vi "SCA-RT_new.vi"() -> ()   [LabVIEW 2016]
uses:
  controls/SCA states.ctl
  control vi/controls/Gate Valve Readback.ctl
  controls/Vertical Rod states.ctl
  controls/Horizontal Rod states.ctl
  controls/GP307 cluster.ctl
  controls/SCA commands.ctl
  controls/SCA Bypass control.ctl
  controls/SCA broadcast status.ctl
  <vilib>/Platform/TimedLoop/XDataNode/timing_clust.ctl
  <vilib>/Platform/TimedLoop/XDataNode/nitl_modes.ctl
  <vilib>/Platform/TimedLoop/XDataNode/wakeup.ctl
  controls/Encoder bit cluster.ctl
  <vilib>/Analysis/baseanly.llb/Mean (DBL).vi
  <vilib>/Instr/_visa.llb/VISA Configure Serial Port (Instr).vi
  <vilib>/Motion/Express/_s/nimc.fb.straightLineMove.startStraightLineMove.axis.modeRelative.0.vi
  <vilib>/Platform/TimedLoop/XDataNode/loadnilvce.vi
  <vilib>/Motion/BlockNode/FB.NIMotion.xnode
  <vilib>/Platform/TimedLoop/XDataNode/XDataNode.xnode
  <vilib>/Platform/TimedLoop/XDataNode/XDNodeRunTimeDep.lvlib
  <vilib>/Analysis/NI_AALBase.lvlib
  <vilib>/NI_Real-Time Target Support.lvlib
panel:
  in  "New sample":i8=1
  in  "Step Window Radius":u8=1
  in  "Rollover Sample":i16=64
  in  "Encoder Offset":i16=160
  out "Bypass error":errorcluster
  out "HV Readback error":errorcluster
  out "SCA command monitor error":errorcluster
  in  "Insert Rod Bypass":bool
  in  "Retract Rod Bypass":bool
  in  "Sample Rod Bypass":bool
  in  "Wheel GV Bypass":bool
  out "Bypass Control":T1
  out "Immersion Lens I set":dbl
  out "Immersion Lens V Set":dbl
  out "SCA Command":T2=enum."Retract insert rod"
  out "Encoder error":errorcluster
  out "Convectron readback error":errorcluster
  out "HV Control error":errorcluster
  out "Rotate Wheel error":errorcluster
  out "Ion Source Vac Cluster":T3
  out "Bellows Vac Cluster":T3
  out "SCA-cRIO error":errorcluster
  out "Insert Rod Status":T4
  out "Retract Rod Status":T4
  out "Sample Rod status":T5
  out "Wheel GV":T6
  out "Raw bits":bool[](array[boolean])
  out "Converted bits":bool[](array[boolean])
  out "Immersion Lens I read":dbl format="%0.2f"
  out "Immersion Lens V read":dbl format="%0.2f"
  out "SCA next state":T7
  out "Extractor I read":dbl
  out "Extractor V read":dbl
  out "Extractor V set":dbl
  out "Cathode V read":dbl
  out "Cathode I read":dbl
  out "Cathode V set":dbl
  out "New Move":dbl
  out "Encoder Destination":dbl
  out "In Range?":bool
  out "Window Limit 2":u32
  out "Window Limit 1":u32
  out "Encoder position":u16
  out "action":string
  out "Vac Readback error":errorcluster
  out "Sample Wheel Convectron":string
  out "Sample Rod UP sensor":bool
  out "Sample Rod DOWN sensor":bool
  out "Rotation done":bool
  out "Insert Rod IN sensor":bool
  out "Insert Rod OUT sensor":bool
  out "Retract Rod IN sensor":bool
  out "Retract Rod OUT sensor":bool
  out "Sensor error":errorcluster
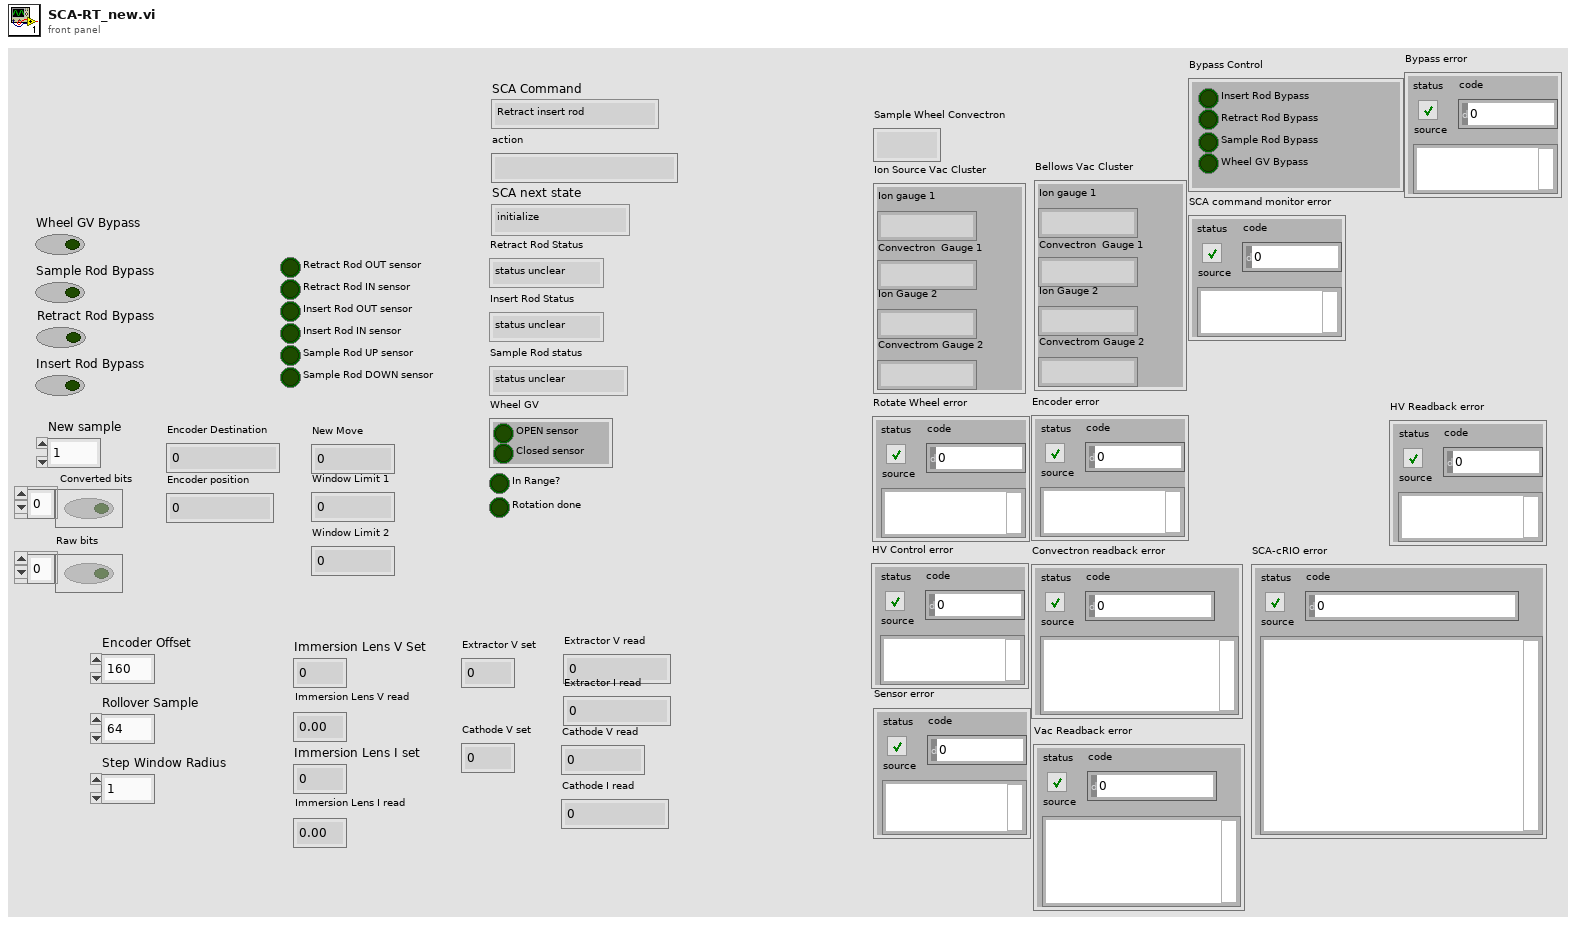
[diagram p1: front panel]
types:
  T1 = typedef "SCA Bypass control.ctl" = cluster{"Insert Rod Bypass":bool, "Retract Rod Bypass":bool, "Sample Rod Bypass":bool, "Wheel GV Bypass":bool}
  T2 = typedef "SCA commands.ctl" = enum16{"Wait", "Shutdown", "Retract insert rod", "Insert insert rod", "Retract retract rod", "Insert retract rod", "Retract sample rod", "Insert sample rod", "Open wheel GV", "Close wheel GV", "Open ion source GV", "Close ion source GV", "Pump out source", "Vent source", "Rotate wheel randomly", "Rotate wheel", "Start random sample change", "Start sample change"}
  T3 = typedef "GP307 cluster.ctl" = cluster{"Ion gauge 1":string, "Convectron  Gauge 1 ":string, "Ion Gauge 2":string, "Convectrom Gauge 2":string}
  T4 = typedef "Horizontal Rod states.ctl" = enum16{"status unclear", "rod in", "rod out"}
  T5 = typedef "Vertical Rod states.ctl" = enum16{"status unclear", "rod down", "rod up"}
  T6 = typedef "Gate Valve Readback.ctl" = cluster{"OPEN sensor":bool, "Closed sensor":bool}
  T7 = typedef "SCA states.ctl" = enum16{"initialize", "wait", "change sample start", "change sample", "check position", "rotate wheel", "sample change complete", "sample rod up", "sample rod down", "retract rod in", "retract rod out", "insert rod in", "insert rod out", "wheel GV open", "wheel GV close", "vent source", "pump source", "shutdown"}
  T8 = typedef "SCA broadcast status.ctl" = enum16{"Waiting", "Changing samples", "Sample change complete", "Failure"}
  T9 = typedef "GV states.ctl" = enum16{"status unclear", "closed", "open"}
  T10 = typedef "XDNodeRunTimeDep.lvlib/timing_clust.ctl" = cluster{"Expected End [f-1]":u64, "Actual End [f-1]":u64, "Finished Late? [f-1]":bool, "Expected End [i-1]":u64, "Actual End [i-1]":u64, "Finished Late? [i-1]":bool, "Expected Start [i]":u64, "Actual Start [i]":u64, "Expected Start [f]":u64, "Actual Start [f]":u64, "Source Name":string, "Structure Name":string, "Period":i64, "Deadline":i64, "Offset":i64, "Start":i64, "Priority":i32, "Timeout":i32, "Mode":T11, "Wakeup Reason":T12, "Error":errorcluster, "Source Type":string, "Secondary Source Type":string, "Global End Time":u64, "Global Start Time":u64, "Frame Duration":u64, "Iteration Duration":u64, "Assigned CPU":i32, "I/O Scan Engine Mode":u32}
  T11 = typedef "XDNodeRunTimeDep.lvlib/nitl_modes.ctl" = enum32{"No Change", "Process missed periods, maintain original phase", "Discard missed periods, maintain original phase", "Process missed periods, ignore original phase", "Discard missed periods, ignore original phase"}
  T12 = typedef "XDNodeRunTimeDep.lvlib/wakeup.ctl" = enum32{"Normal", "Aborted", "Asynchronous wakeup", "Timing source error", "Timed loop error", "Timeout"}
  T13 = typedef "Encoder bit cluster.ctl" = cluster{"MSB":bool, "13th bit":bool, "12th bit":bool, "11th bit":bool, "10th bit":bool, "9th bit":bool, "8th bit":bool, "7th bit":bool, "6th bit":bool, "5th bit":bool, "4th bit":bool, "3rd bit":bool, "2nd bit":bool, "LSB":bool}
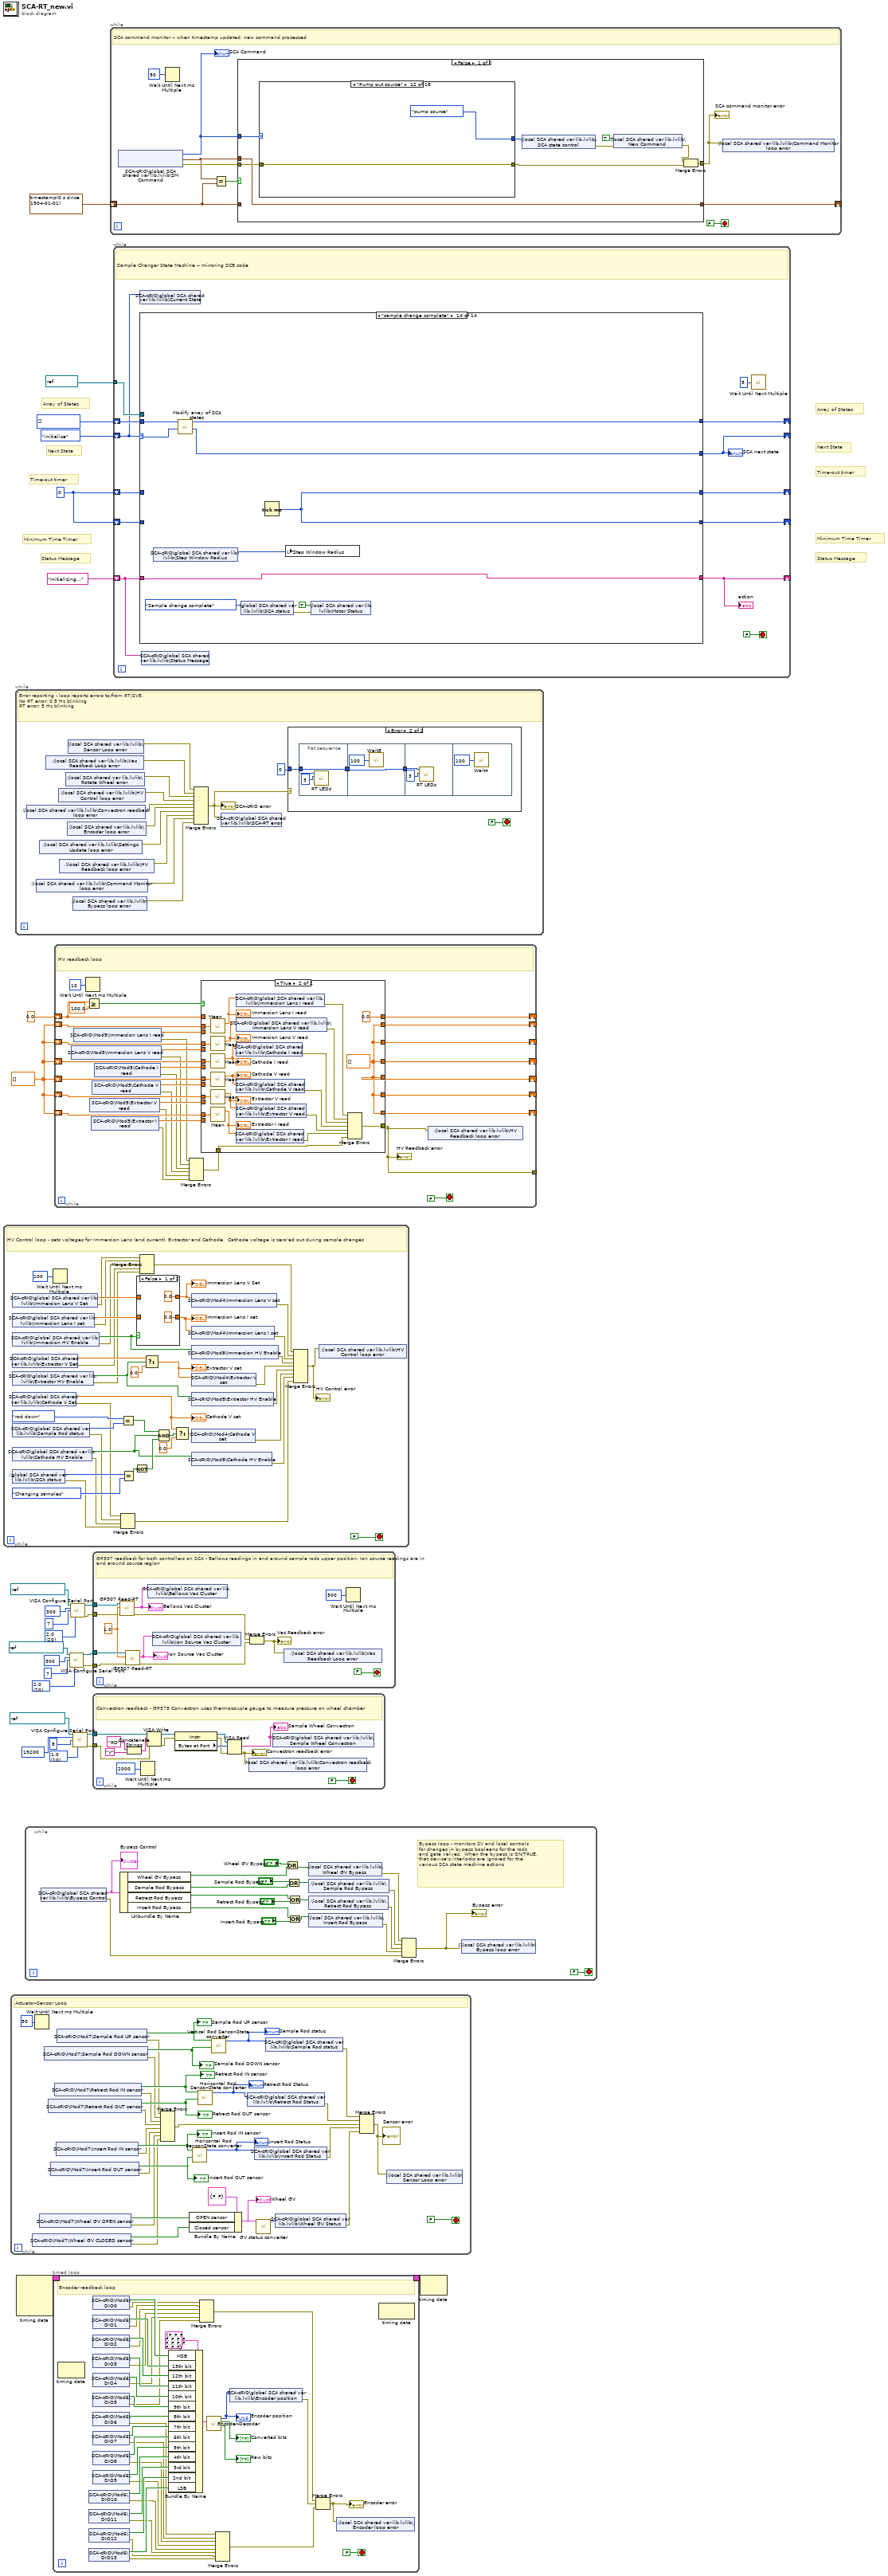
[diagram p0: block diagram]
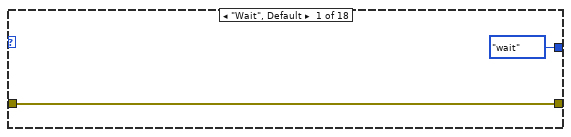
[diagram p2: hidden frame]
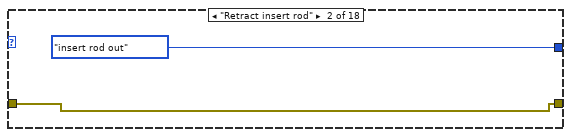
[diagram p3: hidden frame]
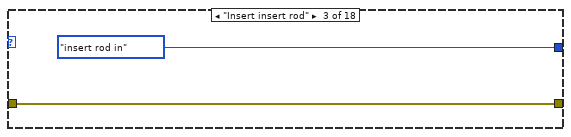
[diagram p4: hidden frame]
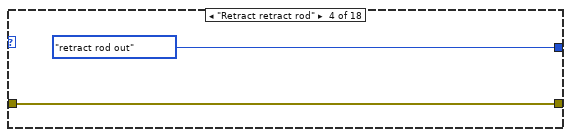
[diagram p5: hidden frame]
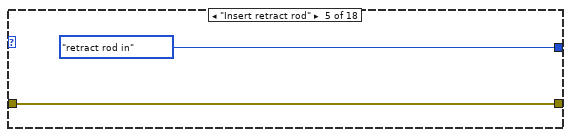
[diagram p6: hidden frame]
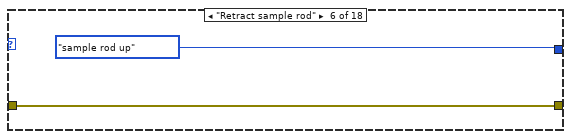
[diagram p7: hidden frame]
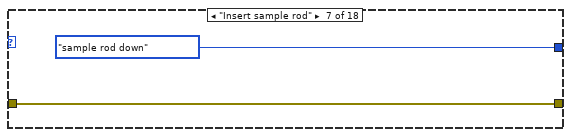
[diagram p8: hidden frame]
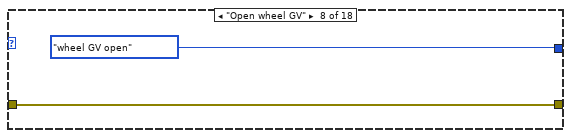
[diagram p9: hidden frame]
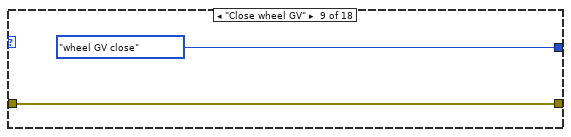
[diagram p10: hidden frame]
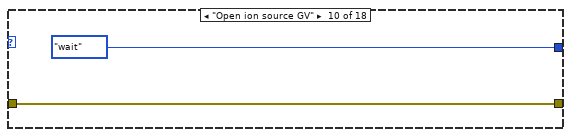
[diagram p11: hidden frame]
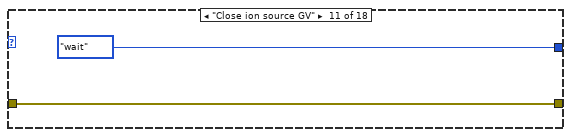
[diagram p12: hidden frame]
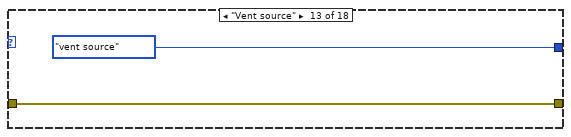
[diagram p13: hidden frame]
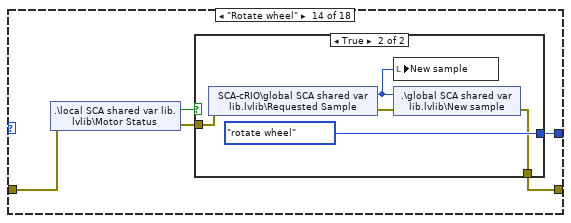
[diagram p14: hidden frame]
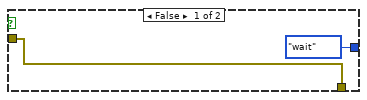
[diagram p15: hidden frame]
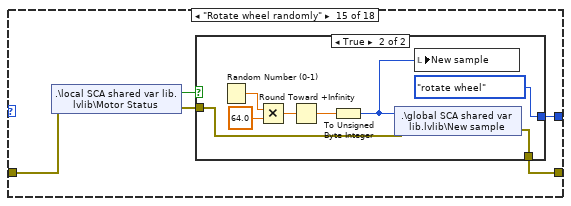
[diagram p16: hidden frame]
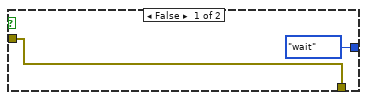
[diagram p17: hidden frame]
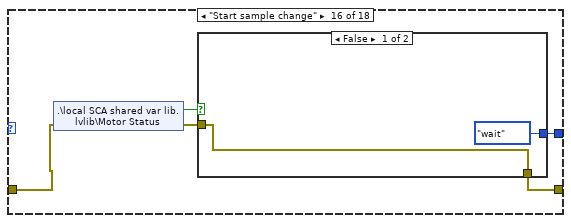
[diagram p18: hidden frame]
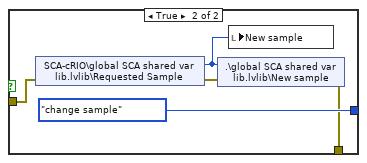
[diagram p19: hidden frame]
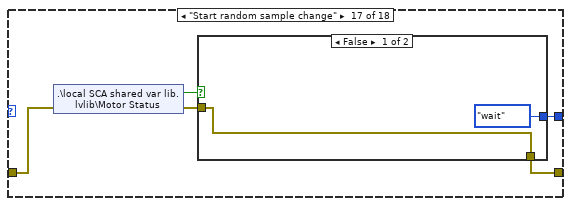
[diagram p20: hidden frame]
diagram:
  w4 = u32 0
  w6 = T7[] [] items=["initialize", "wait", "change sample start", "change sample", "check position", "rotate wheel", "sample change complete", "sample rod up", "sample rod down", "retract rod in", "retract rod out", "insert rod in", "insert rod out", "wheel GV open", "wheel GV close", "vent source", "pump source", "shutdown"]
  w22 = u16 20 items=["1.0"=10, "1.5"=15, "2.0"=20] ("stop bits (10: 1 bit)")
  w26 = u16 10 items=["1.0"=10, "1.5"=15, "2.0"=20] ("stop bits (10: 1 bit)")
  w16 = u16 20 items=["1.0"=10, "1.5"=15, "2.0"=20] ("stop bits (10: 1 bit)")
  w27 = dbl[] []
  # "Status Message"
  # "Array of States"
  # "Next State"
  # "Time-out timer"
  # "Minimum Time Timer"
  # "Status Message"
  # "Array of States"
  # "Next State"
  # "Time-out timer"
  # "Minimum Time Timer"
  n1 = while {
    stop <- FALSE stop-if-true
    # "HV Control loop - sets voltages for Immersion Lens (and current), Extractor and Cathode.  Cathode voltage is zero'ed out during sample changes"
    n2 = shared-variable "SCA-cRIO\\global SCA shared var lib.lvlib\\Immersion Lens V Set"() -> (w61:dbl, error out=w47:errorcluster)  [unwired: 1 in]
    n3 = shared-variable "SCA-cRIO\\global SCA shared var lib.lvlib\\Immersion Lens I set"() -> (w59:dbl, error out=w46:errorcluster)  [unwired: 1 in]
    n4 = shared-variable "SCA-cRIO\\global SCA shared var lib.lvlib\\Immersion HV Enable"() -> (w52:bool, error out=w45:errorcluster)  [unwired: 1 in]
    n5 = shared-variable "SCA-cRIO\\global SCA shared var lib.lvlib\\Extractor V Set"() -> (w57:dbl, error out=w44:errorcluster)  [unwired: 1 in]
    n6 = shared-variable "SCA-cRIO\\global SCA shared var lib.lvlib\\Extractor HV Enable"() -> (w51:bool, error out=w43:errorcluster)  [unwired: 1 in]
    n7 = shared-variable "SCA-cRIO\\global SCA shared var lib.lvlib\\Cathode V Set"() -> (w67:dbl, error out=w39:errorcluster)  [unwired: 1 in]
    "Cathode V set" <- w67
    n8 = shared-variable "SCA-cRIO\\global SCA shared var lib.lvlib\\Sample Rod status"() -> (w63:T5, error out=w40:errorcluster)  [unwired: 1 in]
    n9 = shared-variable "SCA-cRIO\\global SCA shared var lib.lvlib\\Cathode HV Enable"() -> (w53:bool, error out=w41:errorcluster)  [unwired: 1 in]
    n10 = shared-variable ".\\global SCA shared var lib.lvlib\\SCA status"() -> (w49:T8, error out=w42:errorcluster)  [unwired: 1 in]
    n11 = Wait Until Next ms Multiple(millisecond multiple=u32 100) -> ()  [unwired: 1 out]
    n12 = Equal?(x=Vertical_Rod_states."rod down", y=w63) -> (x = y?=w64:bool)
    n13 = Merge Errors(w39, w40, w41, w42) -> (w31:errorcluster)
    n14 = Equal?(x=w49, y=SCA_broadcast_status."Changing samples") -> (x = y?=w48:bool)
    n15 = Not(x=w48) -> (.not. x?=w54:bool)
    n16 = case shown="False" w52 {
      tunnel: [0.0 ("Double") w74] -> w60
      tunnel: w61 -> [_ w74]
      tunnel: w59 -> [_ w73]
      tunnel: [0.0 ("Double") w73] -> w58
      frame False {
      }
      frame True {
      }
    }
    "Immersion Lens V Set" <- w60
    "Immersion Lens I set" <- w58
    n17 = Merge Errors(w47, w46, w45, w44, w43) -> (w30:errorcluster)
    n18 = Select(t=w57, s=w51, f=0.0) -> (s? t:f=w56:dbl)
    "Extractor V set" <- w56
    n19 = Compound Arithmetic op=AND(w64, w53, w54) -> (w68:bool)
    n20 = Select(t=w67, s=w68, f=0.0) -> (s? t:f=w65:dbl)
    n21 = shared-variable "SCA-cRIO\\Mod4\\Immersion Lens V set"(w60) -> (error out=w36:errorcluster)  [unwired: 1 in]
    n22 = shared-variable "SCA-cRIO\\Mod4\\Immersion Lens I set"(w58) -> (error out=w37:errorcluster)  [unwired: 1 in]
    n23 = shared-variable "SCA-cRIO\\Mod8\\Immersion HV Enable"(w52) -> (error out=w38:errorcluster)  [unwired: 1 in]
    n24 = shared-variable "SCA-cRIO\\Mod4\\Extractor V set"(w56) -> (error out=w35:errorcluster)  [unwired: 1 in]
    n25 = shared-variable "SCA-cRIO\\Mod8\\Extractor HV Enable"(w51) -> (error out=w34:errorcluster)  [unwired: 1 in]
    n26 = shared-variable "SCA-cRIO\\Mod4\\Cathode V set"(w65) -> (error out=w33:errorcluster)  [unwired: 1 in]
    n27 = shared-variable "SCA-cRIO\\Mod8\\Cathode HV Enable"(w53) -> (error out=w32:errorcluster)  [unwired: 1 in]
    n28 = Merge Errors(w30, w36, w37, w38, w35, w34, w33, w32, w31) -> (w29:errorcluster)
    "HV Control error" <- w29
    n29 = shared-variable ".\\local SCA shared var lib.lvlib\\HV Control loop error"(w29) -> ()  [unwired: 1 in, 1 out]
  }
  n30 = while {
    stop <- FALSE ("stop") stop-if-true
    # "Actuator-Sensor Loop"
    n31 = shared-variable "SCA-cRIO\\Mod7\\Wheel GV CLOSED sensor"() -> (w100:bool, error out=w79:errorcluster)  [unwired: 1 in]
    n32 = Wait Until Next ms Multiple(millisecond multiple=u32 50) -> ()  [unwired: 1 out]
    n33 = shared-variable "SCA-cRIO\\Mod7\\Wheel GV OPEN sensor"() -> (w99:bool, error out=w78:errorcluster)  [unwired: 1 in]
    n34 = shared-variable "SCA-cRIO\\Mod7\\Sample Rod DOWN sensor"() -> (w96:bool, error out=w82:errorcluster)  [unwired: 1 in]
    "Sample Rod DOWN sensor" <- w96
    n35 = shared-variable "SCA-cRIO\\Mod7\\Retract Rod OUT sensor"() -> (w93:bool, error out=w80:errorcluster)  [unwired: 1 in]
    "Retract Rod OUT sensor" <- w93
    n36 = shared-variable "SCA-cRIO\\Mod7\\Insert Rod OUT sensor"() -> (w91:bool, error out=w77:errorcluster)  [unwired: 1 in]
    "Insert Rod OUT sensor" <- w91
    n37 = shared-variable "SCA-cRIO\\Mod7\\Retract Rod IN sensor"() -> (w94:bool, error out=w81:errorcluster)  [unwired: 1 in]
    "Retract Rod IN sensor" <- w94
    n38 = shared-variable "SCA-cRIO\\Mod7\\Insert Rod IN sensor"() -> (w92:bool, error out=w76:errorcluster)  [unwired: 1 in]
    "Insert Rod IN sensor" <- w92
    n39 = shared-variable "SCA-cRIO\\Mod7\\Sample Rod UP sensor"() -> (w97:bool, error out=w83:errorcluster)  [unwired: 1 in]
    "Sample Rod UP sensor" <- w97
    n40 = Merge Errors(w83, w82, w81, w80, w76, w77, w78, w79) -> (w75:errorcluster)
    n41 = Bundle By Name(cluster=T6 {"OPEN sensor"=FALSE, "Closed sensor"=FALSE} ("Gate Valve"), "OPEN sensor"=w99, "Closed sensor"=w100) -> (w102:T6)
    "Wheel GV" <- w102
    n42 = call "Horizontal Rod Sensor-State converter.vi"("IN Sensor"=w92, "OUT Sensor"=w91) -> ("Status"=w90:T4)  [unwired: 8 in]
    "Insert Rod Status" <- w90
    n43 = call "Horizontal Rod Sensor-State converter.vi"("IN Sensor"=w94, "OUT Sensor"=w93) -> ("Status"=w89:T4)  [unwired: 8 in]
    "Retract Rod Status" <- w89
    n44 = call "Vertical Rod Sensor-State converter.vi"("UP Sensor"=w97, "DOWN Sensor"=w96) -> ("Status"=w95:T5)  [unwired: 8 in]
    "Sample Rod status" <- w95
    n45 = shared-variable "SCA-cRIO\\global SCA shared var lib.lvlib\\Retract Rod Status"(w89) -> (error out=w86:errorcluster)  [unwired: 1 in]
    n46 = shared-variable "SCA-cRIO\\global SCA shared var lib.lvlib\\Insert Rod Status"(w90) -> (error out=w85:errorcluster)  [unwired: 1 in]
    n47 = call "GV status converter.vi"("Gate Valve"=w102) -> ("GV Status"=w98:T9)  [unwired: 10 in]
    n48 = shared-variable "SCA-cRIO\\global SCA shared var lib.lvlib\\Sample Rod status"(w95) -> (error out=w87:errorcluster)  [unwired: 1 in]
    n49 = shared-variable "SCA-cRIO\\global SCA shared var lib.lvlib\\Wheel GV Status"(w98) -> (error out=w84:errorcluster)  [unwired: 1 in]
    n50 = Merge Errors(w87, w86, w75, w85, w84) -> (w88:errorcluster)
    "Sensor error" <- w88
    n51 = shared-variable ".\\local SCA shared var lib.lvlib\\Sensor Loop error"(w88) -> ()  [unwired: 1 in, 1 out]
  }
  n52 = while {
    stop <- FALSE stop-if-true
    # "Error reporting - loop reports errors to/from RT/SVE. \nNo RT error: 0.5 Hz blinking\nRT error: 5 Hz blinking"
    n53 = shared-variable ".\\local SCA shared var lib.lvlib\\Convectron readback loop error"() -> (w110:errorcluster)  [unwired: 1 in, 1 out]
    n54 = shared-variable ".\\local SCA shared var lib.lvlib\\Command Monitor loop error"() -> (w106:errorcluster)  [unwired: 1 in, 1 out]
    n55 = shared-variable ".\\local SCA shared var lib.lvlib\\Settings Update loop error"() -> (w108:errorcluster)  [unwired: 1 in, 1 out]
    n56 = shared-variable ".\\local SCA shared var lib.lvlib\\Vac Readback Loop error"() -> (w115:errorcluster)  [unwired: 1 in, 1 out]
    n57 = shared-variable ".\\local SCA shared var lib.lvlib\\HV Control loop error"() -> (w111:errorcluster)  [unwired: 1 in, 1 out]
    n58 = shared-variable ".\\local SCA shared var lib.lvlib\\HV Readback loop error"() -> (w107:errorcluster)  [unwired: 1 in, 1 out]
    n59 = shared-variable ".\\local SCA shared var lib.lvlib\\Rotate Wheel error"() -> (w112:errorcluster)  [unwired: 1 in, 1 out]
    n60 = shared-variable ".\\local SCA shared var lib.lvlib\\Encoder loop error"() -> (w109:errorcluster)  [unwired: 1 in, 1 out]
    n61 = shared-variable ".\\local SCA shared var lib.lvlib\\Sensor Loop error"() -> (w116:errorcluster)  [unwired: 1 in, 1 out]
    n62 = shared-variable ".\\local SCA shared var lib.lvlib\\Bypass loop error"() -> (w105:errorcluster)  [unwired: 1 in, 1 out]
    n63 = Merge Errors(w116, w115, w112, w111, w110, w109, w108, w107, w106, w105) -> (w114:errorcluster)
    "SCA-cRIO error" <- w114
    n64 = shared-variable "SCA-cRIO\\global SCA shared var lib.lvlib\\SCA-RT error"(w114) -> ()  [unwired: 1 in, 1 out]
    n65 = case shown="Error" w114 {
      tunnel: 0 -> [w120 w128]
      frame No Error {
        n66 = flat-sequence {
          tunnel: w120 -> [w121]
          tunnel: [w121] -> w118
          tunnel: [w123] -> w119
          tunnel: w118 -> [w123]
          tunnel: w119 -> [w125]
          frame #0 {
            n67 = call <vilib>:"RT LEDs.vi"("State"=3, "LED Num"=w121) -> ()  [unwired: 4 in, 2 out]
          }
          frame #1 {
            n68 = call "Wait"("Count(mSec)"=u16 1000) -> ()  [unwired: 1 out]
          }
          frame #2 {
            n69 = call <vilib>:"RT LEDs.vi"("State"=3, "LED Num"=w125) -> ()  [unwired: 4 in, 2 out]
          }
          frame #3 {
            n70 = call "Wait2"("Count(mSec)"=u16 1000) -> ()  [unwired: 1 out]
          }
        }
      }
      frame Error {
        n71 = flat-sequence {
          tunnel: [w131] -> w130
          tunnel: w128 -> [w131]
          tunnel: w130 -> [w133]
          tunnel: [w133] -> w129
          tunnel: w129 -> [w135]
          frame #0 {
            n72 = call <vilib>:"RT LEDs.vi"("State"=3, "LED Num"=w131) -> ()  [unwired: 4 in, 2 out]
          }
          frame #1 {
            n73 = call "Wait3"("Count(mSec)"=u16 100) -> ()  [unwired: 1 out]
          }
          frame #2 {
            n74 = call <vilib>:"RT LEDs.vi"("State"=3, "LED Num"=w135) -> ()  [unwired: 4 in, 2 out]
          }
          frame #3 {
            n75 = call "Wait4"("Count(mSec)"=u16 100) -> ()  [unwired: 1 out]
          }
        }
      }
    }
  }
  n76 = node-c288() -> (w8:T10)  [unwired: 4 in]
  n77 = while {
    stop <- FALSE stop-if-true
    # "Bypass loop - monitors SV and local controls\nfor changes in bypass booleans for the rods \nand gate valves.  When the bypass is ON/TRUE,\nthat device's interlocks are ignored for the \nvarious SCA state machine actions"
    n78 = shared-variable "SCA-cRIO\\global SCA shared var lib.lvlib\\Bypass Control"() -> (w151:T1, error out=w139:errorcluster)  [unwired: 1 in]
    "Bypass Control" <- w151
    n79 = Unbundle By Name(w151) -> ("Wheel GV Bypass"=w148:bool, "Sample Rod Bypass"=w147:bool, "Retract Rod Bypass"=w146:bool, "Insert Rod Bypass"=w145:bool)
    n80 = Or(x="Wheel GV Bypass", y=w148) -> (x .or. y?=w155:bool)
    n81 = Or(x="Sample Rod Bypass", y=w147) -> (x .or. y?=w154:bool)
    n82 = Or(x=w146, y="Retract Rod Bypass") -> (x .or. y?=w152:bool)
    n83 = Or(x=w145, y="Insert Rod Bypass") -> (x .or. y?=w153:bool)
    n84 = shared-variable ".\\local SCA shared var lib.lvlib\\Wheel GV Bypass"(w155) -> (error out=w143:errorcluster)  [unwired: 1 in]
    n85 = shared-variable ".\\local SCA shared var lib.lvlib\\Sample Rod Bypass"(w154) -> (error out=w142:errorcluster)  [unwired: 1 in]
    n86 = shared-variable ".\\local SCA shared var lib.lvlib\\Retract Rod Bypass"(w152) -> (error out=w141:errorcluster)  [unwired: 1 in]
    n87 = shared-variable ".\\local SCA shared var lib.lvlib\\Insert Rod Bypass"(w153) -> (error out=w140:errorcluster)  [unwired: 1 in]
    n88 = Merge Errors(w143, w142, w141, w140, w139) -> (w138:errorcluster)
    "Bypass error" <- w138
    n89 = shared-variable ".\\local SCA shared var lib.lvlib\\Bypass loop error"(w138) -> ()  [unwired: 1 in, 1 out]
  }
  n90 = timed-loop {
    timing: w8 -> [_]
    timing-out: [_] -> w7
    stop <- FALSE stop-if-true
    # "Encoder readback loop"
    n91 = node-c288() -> ()  [unwired: 1 in, 1 out]
    n92 = shared-variable "SCA-cRIO\\Mod6\\DIO10"() -> (w187:bool, error out=w170:errorcluster)  [unwired: 1 in]
    n93 = shared-variable "SCA-cRIO\\Mod6\\DIO11"() -> (w186:bool, error out=w171:errorcluster)  [unwired: 1 in]
    n94 = shared-variable "SCA-cRIO\\Mod6\\DIO12"() -> (w185:bool, error out=w172:errorcluster)  [unwired: 1 in]
    n95 = shared-variable "SCA-cRIO\\Mod6\\DIO13"() -> (w184:bool, error out=w173:errorcluster)  [unwired: 1 in]
    n96 = shared-variable "SCA-cRIO\\Mod6\\DIO0"() -> (w193:bool, error out=w164:errorcluster)  [unwired: 1 in]
    n97 = shared-variable "SCA-cRIO\\Mod6\\DIO1"() -> (w192:bool, error out=w163:errorcluster)  [unwired: 1 in]
    n98 = shared-variable "SCA-cRIO\\Mod6\\DIO2"() -> (w183:bool, error out=w162:errorcluster)  [unwired: 1 in]
    n99 = shared-variable "SCA-cRIO\\Mod6\\DIO3"() -> (w182:bool, error out=w161:errorcluster)  [unwired: 1 in]
    n100 = shared-variable "SCA-cRIO\\Mod6\\DIO4"() -> (w191:bool, error out=w160:errorcluster)  [unwired: 1 in]
    n101 = shared-variable "SCA-cRIO\\Mod6\\DIO5"() -> (w190:bool, error out=w159:errorcluster)  [unwired: 1 in]
    n102 = shared-variable "SCA-cRIO\\Mod6\\DIO6"() -> (w189:bool, error out=w166:errorcluster)  [unwired: 1 in]
    n103 = shared-variable "SCA-cRIO\\Mod6\\DIO7"() -> (w176:bool, error out=w167:errorcluster)  [unwired: 1 in]
    n104 = shared-variable "SCA-cRIO\\Mod6\\DIO8"() -> (w188:bool, error out=w168:errorcluster)  [unwired: 1 in]
    n105 = shared-variable "SCA-cRIO\\Mod6\\DIO9"() -> (w181:bool, error out=w169:errorcluster)  [unwired: 1 in]
    n106 = Bundle By Name(cluster=T13 {"MSB"=FALSE, "13th bit"=FALSE, "12th bit"=FALSE, "11th bit"=FALSE, "10th bit"=FALSE, "9th bit"=FALSE, "8th bit"=FALSE, "7th bit"=FALSE, "6th bit"=FALSE, "5th bit"=FALSE, "4th bit"=FALSE, "3rd bit"=FALSE, "2nd bit"=FALSE, "LSB"=FALSE} ("Cluster"), "MSB"=w193, "13th bit"=w192, "12th bit"=w183, "11th bit"=w182, "10th bit"=w191, "9th bit"=w190, "8th bit"=w189, "7th bit"=w176, "6th bit"=w188, "5th bit"=w181, "4th bit"=w187, "3rd bit"=w186, "2nd bit"=w185, "LSB"=w184) -> (w195:T13)
    n107 = Merge Errors(w164, w163, w162, w161, w160, w159) -> (w158:errorcluster)
    n108 = call "Encoder-Decoder.vi"("Encoder data"=w195) -> ("Raw bits"=→"Raw bits":bool[], "Converted bits"=→"Converted bits":bool[], "Encoder position"=w180:u16)  [unwired: 8 in]
    "Encoder position" <- w180
    n109 = Merge Errors(w166, w167, w168, w169, w170, w171, w172, w173) -> (w165:errorcluster)
    n110 = shared-variable "SCA-cRIO\\global SCA shared var lib.lvlib\\Encoder position"(w180) -> (error out=w174:errorcluster)  [unwired: 1 in]
    n111 = Merge Errors(w158, w174, w165) -> (w175:errorcluster)
    "Encoder error" <- w175
    n112 = shared-variable ".\\local SCA shared var lib.lvlib\\Encoder loop error"(w175) -> ()  [unwired: 1 in, 1 out]
    n113 = node-c288() -> ()  [unwired: 1 in, 1 out]
  }
  n114 = while {
    shift-right: [w222] -> _
    shift-left: 0.0 ("AI1") -> [w225]
    shift-right: [w220] -> _
    shift-left: w27 -> [w219]
    shift-right: [w221] -> _
    shift-left: w27 -> [w218]
    shift-right: [w216] -> _
    shift-left: w27 -> [w215]
    shift-right: [w213] -> _
    shift-left: w27 -> [w212]
    shift-right: [w207] -> _
    shift-left: w27 -> [w210]
    shift-right: [w206] -> _
    shift-left: w27 -> [w211]
    tunnel: [w198] -> _
    stop <- FALSE stop-if-true
    # "HV readback loop"
    n115 = shared-variable "SCA-cRIO\\Mod5\\Immersion Lens V read"() -> (w208:dbl, error out=w204:errorcluster)  [unwired: 1 in]
    n116 = shared-variable "SCA-cRIO\\Mod5\\Immersion Lens I read"() -> (w209:dbl, error out=w205:errorcluster)  [unwired: 1 in]
    n117 = Wait Until Next ms Multiple(millisecond multiple=u32 10) -> ()  [unwired: 1 out]
    n118 = Greater Or Equal?(x=w225, y=100.0) -> (x >= y?=w223:bool)
    n119 = shared-variable "SCA-cRIO\\Mod5\\Extractor V read"() -> (w217:dbl, error out=w201:errorcluster)  [unwired: 1 in]
    n120 = shared-variable "SCA-cRIO\\Mod5\\Extractor I read"() -> (w214:dbl, error out=w200:errorcluster)  [unwired: 1 in]
    n121 = shared-variable "SCA-cRIO\\Mod5\\Cathode V read"() -> (w227:dbl, error out=w202:errorcluster)  [unwired: 1 in]
    n122 = shared-variable "SCA-cRIO\\Mod5\\Cathode I read"() -> (w226:dbl, error out=w203:errorcluster)  [unwired: 1 in]
    n123 = Merge Errors(w205, w204, w203, w202, w201, w200) -> (w199:errorcluster)
    n124 = case shown="True" w223 {
      tunnel: w227 -> [w246 _]
      tunnel: w226 -> [w247 _]
      tunnel: w225 -> [w250 _]
      tunnel: [w249 0.0 ("AI1")] -> w222
      tunnel: [w248 w262] -> w221
      tunnel: [w245 w262] -> w220
      tunnel: w219 -> [w244 w270]
      tunnel: w218 -> [w243 w271]
      tunnel: w217 -> [w242 _]
      tunnel: [w241 w262] -> w216
      tunnel: w215 -> [w240 w269]
      tunnel: w214 -> [w239 _]
      tunnel: [w238 w262] -> w213
      tunnel: w212 -> [w237 w268]
      tunnel: w211 -> [w236 w261]
      tunnel: w210 -> [w235 w260]
      tunnel: w209 -> [w234 _]
      tunnel: w208 -> [w233 _]
      tunnel: [w232 w262] -> w207
      tunnel: [w231 w262] -> w206
      tunnel: w199 -> [w230 w257]
      tunnel: [w230 w251] -> w198
      frame False {
        n125 = Build Array (concatenate)(w234, w235) -> (w232:dbl[])
        n126 = Build Array (concatenate)(w233, w236) -> (w231:dbl[])
        n127 = Build Array (concatenate)(w247, w243) -> (w248:dbl[])
        n128 = Build Array (concatenate)(w246, w244) -> (w245:dbl[])
        n129 = Build Array (concatenate)(w242, w240) -> (w241:dbl[])
        n130 = Build Array (concatenate)(w239, w237) -> (w238:dbl[])
        n131 = Increment(x=w250) -> (x+1=w249:dbl)
      }
      frame True {
        w262 = dbl[] []
        n132 = call-poly <vilib>:"Mean.vi"("X"=w260) -> ("mean"=w259:dbl)  [unwired: 1 out]
        "Immersion Lens I read" <- w259
        n133 = call-poly <vilib>:"Mean.vi"("X"=w261) -> ("mean"=w263:dbl)  [unwired: 1 out]
        "Immersion Lens V read" <- w263
        n134 = call-poly <vilib>:"Mean.vi"("X"=w271) -> ("mean"=w267:dbl)  [unwired: 1 out]
        "Cathode I read" <- w267
        n135 = call-poly <vilib>:"Mean.vi"("X"=w270) -> ("mean"=w266:dbl)  [unwired: 1 out]
        "Cathode V read" <- w266
        n136 = call-poly <vilib>:"Mean.vi"("X"=w269) -> ("mean"=w265:dbl)  [unwired: 1 out]
        "Extractor V read" <- w265
        n137 = call-poly <vilib>:"Mean.vi"("X"=w268) -> ("mean"=w264:dbl)  [unwired: 1 out]
        "Extractor I read" <- w264
        n138 = shared-variable "SCA-cRIO\\global SCA shared var lib.lvlib\\Immersion Lens I read"(w259) -> (error out=w258:errorcluster)  [unwired: 1 in]
        n139 = shared-variable "SCA-cRIO\\global SCA shared var lib.lvlib\\Immersion Lens V read"(w263) -> (error out=w256:errorcluster)  [unwired: 1 in]
        n140 = shared-variable "SCA-cRIO\\global SCA shared var lib.lvlib\\Cathode I read"(w267) -> (error out=w255:errorcluster)  [unwired: 1 in]
        n141 = shared-variable "SCA-cRIO\\global SCA shared var lib.lvlib\\Cathode V read"(w266) -> (error out=w254:errorcluster)  [unwired: 1 in]
        n142 = shared-variable "SCA-cRIO\\global SCA shared var lib.lvlib\\Extractor V read"(w265) -> (error out=w253:errorcluster)  [unwired: 1 in]
        n143 = shared-variable "SCA-cRIO\\global SCA shared var lib.lvlib\\Extractor I read"(w264) -> (error out=w252:errorcluster)  [unwired: 1 in]
        n144 = Merge Errors(w258, w256, w255, w254, w253, w252, w257) -> (w251:errorcluster)
      }
    }
    "HV Readback error" <- w198
    n145 = shared-variable ".\\local SCA shared var lib.lvlib\\HV Readback loop error"(w198) -> ()  [unwired: 1 in, 1 out]
  }
  n146 = call-poly "VISA Configure Serial Port"("VISA resource name"=refnum<visa-resource-name> "ASRL2::INSTR", "baud rate (9600)"=u32 300, "data bits (8)"=u16 7, "stop bits (10: 1 bit)"=w16) -> ("VISA resource name out"=w17:refnum<visa-resource-name>, "error out"=w10:errorcluster)  [unwired: 10 in]
  n147 = call-poly "VISA Configure Serial Port"("VISA resource name"=refnum<visa-resource-name> "ASRL4::INSTR", "baud rate (9600)"=u32 300, "data bits (8)"=u16 7, "stop bits (10: 1 bit)"=w22) -> ("VISA resource name out"=w23:refnum<visa-resource-name>, "error out"=w11:errorcluster)  [unwired: 10 in]
  n148 = call-poly "VISA Configure Serial Port"("VISA resource name"=refnum<visa-resource-name> "ASRL3::INSTR", "baud rate (9600)"=u32 19200, "data bits (8)"=u16 8, "stop bits (10: 1 bit)"=w26) -> ("VISA resource name out"=w12:refnum<visa-resource-name>, "error out"=w9:errorcluster)  [unwired: 10 in]
  n149 = while {
    tunnel: w17 -> [w278]
    tunnel: w23 -> [w281]
    tunnel: w11 -> [w274]
    tunnel: w10 -> [w273]
    stop <- FALSE ("stop 4") stop-if-true
    w277 = 1.0 ("Delay Time (s)")
    # "GP307 readback for both controllers on SCA - Bellows readings in and around sample rods upper position; Ion source readings are in and around source region"
    n150 = call "GP307 Read-RT.vi"("error in (no error)"=w274, "Delay Time (s)"=w277, "VISA Refnum in"=w281) -> ("error out"=w279:errorcluster, "GP307 output"=w280:T3)  [unwired: 6 in, 1 out]
    "Bellows Vac Cluster" <- w280
    n151 = call "GP307 Read-RT.vi"("error in (no error)"=w273, "Delay Time (s)"=w277, "VISA Refnum in"=w278) -> ("error out"=w275:errorcluster, "GP307 output"=w276:T3)  [unwired: 6 in, 1 out]
    "Ion Source Vac Cluster" <- w276
    n152 = shared-variable "SCA-cRIO\\global SCA shared var lib.lvlib\\Bellows Vac Cluster"(w280) -> ()  [unwired: 1 in, 1 out]
    n153 = shared-variable "SCA-cRIO\\global SCA shared var lib.lvlib\\Ion Source Vac Cluster"(w276) -> ()  [unwired: 1 in, 1 out]
    n154 = Merge Errors(w279, w275) -> (w282:errorcluster)
    "Vac Readback error" <- w282
    n155 = shared-variable ".\\local SCA shared var lib.lvlib\\Vac Readback Loop error"(w282) -> ()  [unwired: 1 in, 1 out]
    n156 = Wait Until Next ms Multiple(millisecond multiple=u32 500) -> ()  [unwired: 1 out]
  }
  n157 = while {
    tunnel: w12 -> [w291]
    tunnel: w9 -> [w285]
    stop <- FALSE ("stop 3") stop-if-true
    # "Convectron readback - GP375 Convectron uses thermocouple gauge to measure pressure on wheel chamber"
    n158 = Concatenate Strings("RD" ("write buffer 2"), "\r") -> (w298:string)
    n159 = Wait Until Next ms Multiple(millisecond multiple=u32 2000) -> ()  [unwired: 1 out]
    n160 = VISA Write(VISA resource name=w291, write buffer=w298, error in (no error)=w285) -> (VISA resource name out=w292:refnum<visa-resource-name>, error out=w288:errorcluster)  [unwired: 1 out]
    n161 = property class="Instr"(reference=w292, error in=w288) -> (reference out=w293:refnum<visa-resource-name>, error out=w287:errorcluster, "Bytes at Port"=w294:u32)
    n162 = VISA Read(VISA resource name=w293, byte count=w294, error in (no error)=w287) -> (read buffer=w289:string, error out=w286:errorcluster)  [unwired: 2 out]
    "Sample Wheel Convectron" <- w289
    "Convectron readback error" <- w286
    n163 = shared-variable ".\\local SCA shared var lib.lvlib\\Convectron readback loop error"(w286) -> ()  [unwired: 1 in, 1 out]
    n164 = shared-variable "SCA-cRIO\\global SCA shared var lib.lvlib\\Sample Wheel Convectron"(w289) -> ()  [unwired: 1 in, 1 out]
  }
  n165 = while {
    shift-right: [w305] -> _
    shift-left: timestamp(0 s since 1904-01-01) -> [w304]
    stop <- FALSE stop-if-true
    # "SCA command monitor -- when timestamp updated, new command processed"
    n166 = shared-variable "SCA-cRIO\\global SCA shared var lib.lvlib\\SM Command"() -> (w301:T2, error out=w300:errorcluster, w306:timestamp)  [unwired: 1 in]
    "SCA Command" <- w301
    n167 = Wait Until Next ms Multiple(millisecond multiple=u32 50) -> ()  [unwired: 1 out]
    n168 = Equal?(x=w306, y=w304) -> (x = y?=w307:bool)
    n169 = case shown="False" w307 {
      tunnel: w306 -> [w316 _]
      tunnel: [w316 w400] -> w305
      tunnel: w304 -> [_ w400]
      tunnel: w301 -> [w315 _]
      tunnel: w300 -> [w311 w399]
      tunnel: [w308 w399] -> w299
      frame False {
        n170 = case shown="\"Pump out source\"" w315 {
          tunnel: [SCA_states."wait" ("SC2 state") SCA_states."insert rod out" ("SC2 state") SCA_states."insert rod in" ("SC2 state") SCA_states."retract rod out" ("SC2 state") SCA_states."retract rod in" ("SC2 state") SCA_states."sample rod up" ("SC2 state") SCA_states."sample rod down" ("SC2 state") SCA_states."wheel GV open" ("SC2 state") SCA_states."wheel GV close" ("SC2 state") SCA_states."wait" ("SC2 state") SCA_states."wait" ("SC2 state") SCA_states."pump source" ("SC2 state") SCA_states."vent source" ("SC2 state") w347 w359 w374 w385 SCA_states."initialize" ("SC2 state")] -> w314
          tunnel: w311 -> [w318 w319 w321 w323 w325 w327 w329 w331 w333 w335 w337 w339 w341 w345 w357 w372 w384 w398]
          tunnel: [w318 w319 w321 w323 w325 w327 w329 w331 w333 w335 w337 w339 w341 w343 w355 w370 w383 w398] -> w310
          frame "Wait", Default {
          }
          frame "Retract insert rod" {
          }
          frame "Insert insert rod" {
          }
          frame "Retract retract rod" {
          }
          frame "Insert retract rod" {
          }
          frame "Retract sample rod" {
          }
          frame "Insert sample rod" {
          }
          frame "Open wheel GV" {
          }
          frame "Close wheel GV" {
          }
          frame "Open ion source GV" {
          }
          frame "Close ion source GV" {
          }
          frame "Pump out source" {
          }
          frame "Vent source" {
          }
          frame "Rotate wheel" {
            n171 = shared-variable ".\\local SCA shared var lib.lvlib\\Motor Status"(error in=w345) -> (w346:bool, error out=w344:errorcluster)
            n172 = case shown="True" w346 {
              tunnel: [SCA_states."wait" ("SC2 state") SCA_states."rotate wheel" ("SC2 state")] -> w347
              tunnel: w344 -> [w348 w353]
              tunnel: [w348 w351] -> w343
              frame False {
              }
              frame True {
                n173 = shared-variable "SCA-cRIO\\global SCA shared var lib.lvlib\\Requested Sample"(error in=w353) -> (w350:u8, error out=w352:errorcluster)
                n174 = local write "New sample"(w350) -> ()
                n175 = shared-variable ".\\global SCA shared var lib.lvlib\\New sample"(w350, error in=w352) -> (error out=w351:errorcluster)
              }
            }
          }
          frame "Rotate wheel randomly" {
            n176 = shared-variable ".\\local SCA shared var lib.lvlib\\Motor Status"(error in=w357) -> (w358:bool, error out=w356:errorcluster)
            n177 = case shown="True" w358 {
              tunnel: [SCA_states."wait" ("SC2 state") SCA_states."rotate wheel" ("SC2 state")] -> w359
              tunnel: w356 -> [w360 w364]
              tunnel: [w360 w363] -> w355
              frame False {
              }
              frame True {
                n178 = Random Number (0-1)() -> (number: 0 to 1=w367:dbl)
                n179 = Multiply(x=w367, y=64.0) -> (x*y=w365:dbl)
                n180 = Round Toward +Infinity(x=w365) -> (ceil(x): smallest int >= x=w368:dbl)
                n181 = To Unsigned Byte Integer(number=w368) -> (unsigned 8bit integer=w362:u8)
                n182 = shared-variable ".\\global SCA shared var lib.lvlib\\New sample"(w362, error in=w364) -> (error out=w363:errorcluster)
                n183 = local write "New sample"(w362) -> ()
              }
            }
          }
          frame "Start sample change" {
            n184 = shared-variable ".\\local SCA shared var lib.lvlib\\Motor Status"(error in=w372) -> (w373:bool, error out=w371:errorcluster)
            n185 = case shown="False" w373 {
              tunnel: [SCA_states."wait" ("SC2 state") SCA_states."change sample" ("SC2 state")] -> w374
              tunnel: w371 -> [w375 w380]
              tunnel: [w375 w378] -> w370
              frame False {
              }
              frame True {
                n186 = shared-variable "SCA-cRIO\\global SCA shared var lib.lvlib\\Requested Sample"(error in=w380) -> (w377:u8, error out=w379:errorcluster)
                n187 = shared-variable ".\\global SCA shared var lib.lvlib\\New sample"(w377, error in=w379) -> (error out=w378:errorcluster)
                n188 = local write "New sample"(w377) -> ()
              }
            }
          }
          frame "Start random sample change" {
            n189 = shared-variable ".\\local SCA shared var lib.lvlib\\Motor Status"(error in=w384) -> (w386:bool, error out=w382:errorcluster)
            n190 = case shown="False" w386 {
              tunnel: [SCA_states."wait" ("SC2 state") SCA_states."change sample" ("SC2 state")] -> w385
              tunnel: [w387 w391] -> w383
              tunnel: w382 -> [w387 w390]
              frame False {
              }
              frame True {
                n191 = Random Number (0-1)() -> (number: 0 to 1=w394:dbl)
                n192 = Multiply(x=w394, y=64.0) -> (x*y=w392:dbl)
                n193 = Round Toward +Infinity(x=w392) -> (ceil(x): smallest int >= x=w395:dbl)
                n194 = To Unsigned Byte Integer(number=w395) -> (unsigned 8bit integer=w389:u8)
                n195 = local write "New sample"(w389) -> ()
                n196 = shared-variable ".\\global SCA shared var lib.lvlib\\New sample"(w389, error in=w390) -> (error out=w391:errorcluster)
              }
            }
          }
          frame "Shutdown" {
          }
        }
        n197 = shared-variable ".\\local SCA shared var lib.lvlib\\SCA state control"(w314) -> (error out=w312:errorcluster)  [unwired: 1 in]
        n198 = shared-variable ".\\local SCA shared var lib.lvlib\\New Command"(TRUE ("New Command?"), error in=w312) -> (error out=w309:errorcluster)
        n199 = Merge Errors(w309, w310) -> (w308:errorcluster)
      }
      frame True {
      }
    }
    "SCA command monitor error" <- w299
    n200 = shared-variable ".\\local SCA shared var lib.lvlib\\Command Monitor loop error"(w299) -> ()  [unwired: 1 in, 1 out]
  }
  n201 = while {
    shift-right: [w401] -> _
    shift-left: SCA_states."initialize" ("SC2 state") -> [w402]
    shift-right: [w405] -> _
    shift-left: w6 -> [w411]
    shift-right: [w409] -> _
    shift-left: w4 -> [w410]
    shift-right: [w403] -> _
    shift-left: "Initializing..." -> [w406]
    shift-right: [w407] -> _
    shift-left: w4 -> [w408]
    tunnel: refnum<k21> "Axis 1" ("resource") -> [w412]
    stop <- FALSE ("stop 2") stop-if-true
    # "Sample Changer State Machine -- mirroring SCB code"
    n202 = shared-variable "SCA-cRIO\\global SCA shared var lib.lvlib\\Current State"(w402) -> ()  [unwired: 1 in, 1 out]
    n203 = case shown="\"sample change complete\"" w402 {
      selector: w402 -> [_ _ w456 w492 w557 w588 w657 w724 w755 w829 w856 _ w917 w1034]
      tunnel: w412 -> [_ _ _ _ _ _ _ _ _ _ _ w879 w913 _]
      tunnel: [SCA_states."wait" ("SC2 state") w434 w461 w488 w552 w583 w652 w719 w750 w825 w855 w871 w914 w1032] -> w401
      tunnel: w411 -> [w426 _ w458 w494 w558 w589 w658 w725 w756 w830 w858 w872 w912 w1035]
      tunnel: w410 -> [w429 _ w457 w490 w555 w585 w655 w722 w752 w827 _ w862 w909 _]
      tunnel: [w429 w433 w457 w490 w555 w585 w655 w722 w752 w827 w859 w862 w915 w1038] -> w409
      tunnel: [w426 w435 w460 w487 w551 w582 w651 w718 w751 w824 w857 w872 w911 w1033] -> w405
      tunnel: w406 -> [w427 _ _ _ _ _ _ _ _ _ w854 _ _ w1031]
      tunnel: [w427 "Waiting on command" ("t") w462 w491 w554 w586 w654 w721 w753 w823 w854 "rotating wheel" ("t") w910 w1031] -> w403
      tunnel: w408 -> [w430 _ w463 w493 w556 w587 w656 w723 w754 w828 _ w874 w906 _]
      tunnel: [w430 w433 w459 w489 w553 w584 w653 w720 w749 w826 w859 w874 w916 w1038] -> w407
      frame "initialize" {
        w415 = i16 160 ("Encoder Offset")
        w416 = i16 64 ("Rollover Sample")
        w417 = u8 1 ("Step Window Radius")
        n204 = shared-variable ".\\local SCA shared var lib.lvlib\\Motor Status"(TRUE ("Motor Status")) -> ()  [unwired: 1 in, 1 out]
        n205 = shared-variable ".\\global SCA shared var lib.lvlib\\SCA status"(SCA_broadcast_status."Waiting") -> ()  [unwired: 1 in, 1 out]
        n206 = local write "New sample"(i8 1 ("New sample")) -> ()
        n207 = shared-variable ".\\global SCA shared var lib.lvlib\\Rotate Wheel Minimum Time"(u16 1000 ("Rotate Wheel Minimum Time")) -> ()  [unwired: 1 in, 1 out]
        n208 = shared-variable "SCA-cRIO\\global SCA shared var lib.lvlib\\Step Window Radius"(w417) -> ()  [unwired: 1 in, 1 out]
        n209 = local write "Step Window Radius"(w417) -> ()
        n210 = shared-variable ".\\global SCA shared var lib.lvlib\\Retract Rod Timeout"(u32 10000 ("Retract Rod Timeout")) -> ()  [unwired: 1 in, 1 out]
        n211 = shared-variable ".\\global SCA shared var lib.lvlib\\Wheel GV Timeout"(10000 ("Wheel GV Timeout")) -> ()  [unwired: 1 in, 1 out]
        n212 = shared-variable "SCA-cRIO\\global SCA shared var lib.lvlib\\Rollover Sample"(w416) -> ()  [unwired: 1 in, 1 out]
        n213 = local write "Rollover Sample"(w416) -> ()
        n214 = shared-variable ".\\global SCA shared var lib.lvlib\\Rotate Wheel timeout"(u32 30000 ("Rotate Wheel timeout")) -> ()  [unwired: 1 in, 1 out]
        n215 = shared-variable ".\\global SCA shared var lib.lvlib\\Sample Rod Timeout"(u32 10000 ("Sample Rod Timeout")) -> ()  [unwired: 1 in, 1 out]
        n216 = shared-variable ".\\global SCA shared var lib.lvlib\\Insert Rod Timeout"(u32 10000 ("Insert Rod Timeout")) -> ()  [unwired: 1 in, 1 out]
        n217 = local write "Encoder Offset"(w415) -> ()
        n218 = shared-variable "SCA-cRIO\\global SCA shared var lib.lvlib\\Encoder Offset"(w415) -> ()  [unwired: 1 in, 1 out]
      }
      frame "wait", Default {
        n219 = shared-variable ".\\local SCA shared var lib.lvlib\\New Command"() -> (w432:bool)  [unwired: 1 in, 1 out]
        n220 = case shown="True" w432 {
          tunnel: [w437 w440] -> w435
          frame False {
            w437 = T7[] [enum."wait"] items=["initialize", "wait", "change sample start", "change sample", "check position", "rotate wheel", "sample change complete", "sample rod up", "sample rod down", "retract rod in", "retract rod out", "insert rod in", "insert rod out", "wheel GV open", "wheel GV close", "vent source", "pump source", "shutdown"]
          }
          frame True {
            n221 = shared-variable ".\\local SCA shared var lib.lvlib\\SCA state control"() -> (w439:T7)  [unwired: 1 in, 1 out]
            n222 = case shown="\"pump source\"" w439 {
              tunnel: [w441 w442 w443 w444 w445 w446 w447 w448 w449 w450 w451 w452 w453 w454] -> w440
              frame "wheel GV close" {
                w441 = T7[] [enum."wheel GV close", enum."wait"] items=["initialize", "wait", "change sample start", "change sample", "check position", "rotate wheel", "sample change complete", "sample rod up", "sample rod down", "retract rod in", "retract rod out", "insert rod in", "insert rod out", "wheel GV open", "wheel GV close", "vent source", "pump source", "shutdown"]
              }
              frame "wheel GV open" {
                w442 = T7[] [enum."wheel GV open", enum."wait"] items=["initialize", "wait", "change sample start", "change sample", "check position", "rotate wheel", "sample change complete", "sample rod up", "sample rod down", "retract rod in", "retract rod out", "insert rod in", "insert rod out", "wheel GV open", "wheel GV close", "vent source", "pump source", "shutdown"]
              }
              frame "sample rod up" {
                w443 = T7[] [enum."sample rod up", enum."wait"] items=["initialize", "wait", "change sample start", "change sample", "check position", "rotate wheel", "sample change complete", "sample rod up", "sample rod down", "retract rod in", "retract rod out", "insert rod in", "insert rod out", "wheel GV open", "wheel GV close", "vent source", "pump source", "shutdown"]
              }
              frame "sample rod down" {
                w444 = T7[] [enum."sample rod down", enum."wait"] items=["initialize", "wait", "change sample start", "change sample", "check position", "rotate wheel", "sample change complete", "sample rod up", "sample rod down", "retract rod in", "retract rod out", "insert rod in", "insert rod out", "wheel GV open", "wheel GV close", "vent source", "pump source", "shutdown"]
              }
              frame "retract rod in" {
                w445 = T7[] [enum."retract rod in", enum."wait"] items=["initialize", "wait", "change sample start", "change sample", "check position", "rotate wheel", "sample change complete", "sample rod up", "sample rod down", "retract rod in", "retract rod out", "insert rod in", "insert rod out", "wheel GV open", "wheel GV close", "vent source", "pump source", "shutdown"]
              }
              frame "retract rod out" {
                w446 = T7[] [enum."retract rod out", enum."wait"] items=["initialize", "wait", "change sample start", "change sample", "check position", "rotate wheel", "sample change complete", "sample rod up", "sample rod down", "retract rod in", "retract rod out", "insert rod in", "insert rod out", "wheel GV open", "wheel GV close", "vent source", "pump source", "shutdown"]
              }
              frame "insert rod in" {
                w447 = T7[] [enum."insert rod in", enum."wait"] items=["initialize", "wait", "change sample start", "change sample", "check position", "rotate wheel", "sample change complete", "sample rod up", "sample rod down", "retract rod in", "retract rod out", "insert rod in", "insert rod out", "wheel GV open", "wheel GV close", "vent source", "pump source", "shutdown"]
              }
              frame "insert rod out" {
                w448 = T7[] [enum."insert rod out", enum."wait"] items=["initialize", "wait", "change sample start", "change sample", "check position", "rotate wheel", "sample change complete", "sample rod up", "sample rod down", "retract rod in", "retract rod out", "insert rod in", "insert rod out", "wheel GV open", "wheel GV close", "vent source", "pump source", "shutdown"]
              }
              frame "rotate wheel" {
                w449 = T7[] [enum."retract rod out", enum."insert rod out", enum."check position", enum."wait"] items=["initialize", "wait", "change sample start", "change sample", "check position", "rotate wheel", "sample change complete", "sample rod up", "sample rod down", "retract rod in", "retract rod out", "insert rod in", "insert rod out", "wheel GV open", "wheel GV close", "vent source", "pump source", "shutdown"]
              }
              frame "change sample" {
                w450 = T7[] [enum."change sample start", enum."sample rod up", enum."retract rod in", enum."retract rod out", enum."check position", enum."insert rod in", enum."insert rod out", enum."sample rod down", enum."sample change complete", enum."wait"] items=["initialize", "wait", "change sample start", "change sample", "check position", "rotate wheel", "sample change complete", "sample rod up", "sample rod down", "retract rod in", "retract rod out", "insert rod in", "insert rod out", "wheel GV open", "wheel GV close", "vent source", "pump source", "shutdown"]
              }
              frame "vent source" {
                w451 = T7[] [enum."sample rod up", enum."retract rod in", enum."retract rod out", enum."insert rod out", enum."wheel GV close", enum."wait"] items=["initialize", "wait", "change sample start", "change sample", "check position", "rotate wheel", "sample change complete", "sample rod up", "sample rod down", "retract rod in", "retract rod out", "insert rod in", "insert rod out", "wheel GV open", "wheel GV close", "vent source", "pump source", "shutdown"]
              }
              frame "pump source" {
                w452 = T7[] [enum."wheel GV open", enum."sample rod up", enum."check position", enum."insert rod in", enum."insert rod out", enum."sample rod down", enum."wait"] items=["initialize", "wait", "change sample start", "change sample", "check position", "rotate wheel", "sample change complete", "sample rod up", "sample rod down", "retract rod in", "retract rod out", "insert rod in", "insert rod out", "wheel GV open", "wheel GV close", "vent source", "pump source", "shutdown"]
              }
              frame "wait", Default {
                w453 = T7[] [enum."wait"] items=["initialize", "wait", "change sample start", "change sample", "check position", "rotate wheel", "sample change complete", "sample rod up", "sample rod down", "retract rod in", "retract rod out", "insert rod in", "insert rod out", "wheel GV open", "wheel GV close", "vent source", "pump source", "shutdown"]
              }
              frame "shutdown" {
                w454 = T7[] [enum."sample rod up", enum."retract rod in", enum."retract rod out", enum."wheel GV close", enum."wait"] items=["initialize", "wait", "change sample start", "change sample", "check position", "rotate wheel", "sample change complete", "sample rod up", "sample rod down", "retract rod in", "retract rod out", "insert rod in", "insert rod out", "wheel GV open", "wheel GV close", "vent source", "pump source", "shutdown"]
              }
            }
            n223 = shared-variable ".\\local SCA shared var lib.lvlib\\New Command"(FALSE ("New Command?")) -> ()  [unwired: 1 in, 1 out]
          }
        }
        n224 = Index Array(array=w435, index=0) -> (element=w434:T7)
        n225 = Tick Count (ms)() -> (millisecond timer value=w433:u32)
      }
      frame "wheel GV open" {
        n226 = flat-sequence {
          tunnel: [w469] -> w455
          tunnel: [w472] -> w466
          tunnel: w455 -> [w472]
          frame #0 {
            n227 = shared-variable "SCA-cRIO\\Mod8\\Wheel GV Actuator"(TRUE ("sc gate valve")) -> (error out=w469:errorcluster)  [unwired: 1 in]
          }
          frame #1 {
            n228 = Wait (ms)(milliseconds to wait=u32 200) -> ()  [unwired: 1 out]
          }
        }
        n229 = shared-variable ".\\local SCA shared var lib.lvlib\\Wheel GV Bypass"() -> (w468:bool)  [unwired: 1 in, 1 out]
        n230 = shared-variable "SCA-cRIO\\global SCA shared var lib.lvlib\\Wheel GV Status"(error in=w466) -> (w465:enum16{"status unclear", "closed", "open"})  [unwired: 1 out]
        n231 = Select(t=enum16{"status unclear", "closed", "open"}."open" ("x"), s=w468, f=w465) -> (s? t:f=w464:enum16{"status unclear", "closed", "open"})
        n232 = case shown="\"open\"" w464 {
          tunnel: w463 -> [w479 _]
          tunnel: w458 -> [w478 w486]
          tunnel: w456 -> [w477 w485]
          tunnel: [w476 w484] -> w460
          tunnel: [w475 w483] -> w461
          tunnel: [w474 w482] -> w459
          tunnel: [w473 "wheel GV opened" ("Status Message")] -> w462
          frame "status unclear", "closed", Default {
            n233 = shared-variable ".\\global SCA shared var lib.lvlib\\Wheel GV Timeout"() -> (w480:u32)  [unwired: 1 in, 1 out]
            n234 = call "SCA state Transition Timeout Check.vi"("Start Time"=w479, "Timeout limit"=w480, "Current State In"=w477, "Modified Array of states in"=w478) -> ("Status Message"=w473:string, "millisecond timer value out"=w474:u32, "Next State"=w475:T7, "Modified Array of states out"=w476:T7[])  [unwired: 4 in]
          }
          frame "open" {
            n235 = call "Modify array of SCA states.vi"("Current State"=w485, "Array of states to process"=w486) -> ("Next State"=w483:T7, "Modified Array of states"=w484:T7[])  [unwired: 7 in]
            n236 = Tick Count (ms)() -> (millisecond timer value=w482:u32)
          }
        }
      }
      frame "wheel GV close" {
        n237 = shared-variable "SCA-cRIO\\global SCA shared var lib.lvlib\\Retract Rod Status"() -> (w505:T4)  [unwired: 1 in, 1 out]
        n238 = shared-variable "SCA-cRIO\\global SCA shared var lib.lvlib\\Insert Rod Status"() -> (w503:T4)  [unwired: 1 in, 1 out]
        n239 = shared-variable ".\\local SCA shared var lib.lvlib\\Retract Rod Bypass"() -> (w499:bool)  [unwired: 1 in, 1 out]
        n240 = shared-variable ".\\local SCA shared var lib.lvlib\\Insert Rod Bypass"() -> (w501:bool)  [unwired: 1 in, 1 out]
        n241 = Equal?(x=w503, y=Horizontal_Rod_states."rod out" ("Enum")) -> (x = y?=w502:bool)
        n242 = Equal?(x=w505, y=Horizontal_Rod_states."rod out" ("Enum")) -> (x = y?=w500:bool)
        n243 = Or(x=w501, y=w502) -> (x .or. y?=w498:bool)
        n244 = Or(x=w499, y=w500) -> (x .or. y?=w497:bool)
        n245 = Build Array(w498, w497) -> (w495:bool[])
        n246 = And Array Elements(Boolean array=w495) -> (logical AND=w496:bool)
        n247 = case shown="True" w496 {
          tunnel: w495 -> [w514 _]
          tunnel: w494 -> [w510 w529]
          tunnel: w492 -> [_ w528]
          tunnel: w493 -> [_ w527]
          tunnel: ["wheel GV interlocks not satisfied" ("Status Message") w526] -> w491
          tunnel: [w507 w525] -> w489
          tunnel: [w508 w524] -> w488
          tunnel: [w509 w523] -> w487
          frame False {
            n248 = Search 1D Array(1D array=w514, element=FALSE) -> (index of element=w512:i32)  [unwired: 1 in]
            n249 = case shown="0, Default" w512 {
              tunnel: w510 -> [w515 w522]
              tunnel: [w517 w520] -> w509
              tunnel: [w516 w519] -> w508
              frame 0, Default {
                w516 = SCA_states."insert rod out" ("SC2 state")
                n250 = Insert Into Array(array=w515, index=0, new element=w516) -> (w517:T7[])
              }
              frame 1 {
                w519 = SCA_states."retract rod out" ("SC2 state")
                n251 = Insert Into Array(array=w522, index=0, new element=w519) -> (w520:T7[])
              }
            }
            n252 = Tick Count (ms)() -> (millisecond timer value=w507:u32)
          }
          frame True {
            n253 = shared-variable "SCA-cRIO\\Mod8\\Wheel GV Actuator"(FALSE ("sc gate valve")) -> (error out=w532:errorcluster)  [unwired: 1 in]
            n254 = shared-variable ".\\local SCA shared var lib.lvlib\\Wheel GV Bypass"() -> (w535:bool)  [unwired: 1 in, 1 out]
            n255 = shared-variable "SCA-cRIO\\global SCA shared var lib.lvlib\\Wheel GV Status"(error in=w532) -> (w531:enum16{"status unclear", "closed", "open"})  [unwired: 1 out]
            n256 = Select(t=enum16{"status unclear", "closed", "open"}."closed" ("x"), s=w535, f=w531) -> (s? t:f=w530:enum16{"status unclear", "closed", "open"})
            n257 = case shown="\"status unclear\", \"open\", Default" w530 {
              tunnel: w527 -> [w542 _]
              tunnel: w529 -> [w541 w549]
              tunnel: w528 -> [w540 w548]
              tunnel: [w539 w547] -> w523
              tunnel: [w538 w546] -> w524
              tunnel: [w537 w545] -> w525
              tunnel: [w536 "wheel GV closed" ("Status Message")] -> w526
              frame "status unclear", "open", Default {
                n258 = shared-variable ".\\global SCA shared var lib.lvlib\\Wheel GV Timeout"() -> (w543:u32)  [unwired: 1 in, 1 out]
                n259 = call "SCA state Transition Timeout Check.vi"("Start Time"=w542, "Timeout limit"=w543, "Current State In"=w540, "Modified Array of states in"=w541) -> ("Status Message"=w536:string, "millisecond timer value out"=w537:u32, "Next State"=w538:T7, "Modified Array of states out"=w539:T7[])  [unwired: 4 in]
              }
              frame "closed" {
                n260 = call "Modify array of SCA states.vi"("Current State"=w548, "Array of states to process"=w549) -> ("Next State"=w546:T7, "Modified Array of states"=w547:T7[])  [unwired: 7 in]
                n261 = Tick Count (ms)() -> (millisecond timer value=w545:u32)
              }
            }
          }
        }
      }
      frame "sample rod up" {
        n262 = flat-sequence {
          tunnel: [w564] -> w550
          tunnel: [w567] -> w563
          tunnel: w550 -> [w567]
          frame #0 {
            n263 = shared-variable "SCA-cRIO\\Mod8\\Sample Rod Actuator"(FALSE ("Sample Rod Actuator")) -> (error out=w564:errorcluster)  [unwired: 1 in]
          }
          frame #1 {
            n264 = Wait (ms)(milliseconds to wait=u32 500) -> ()  [unwired: 1 out]
          }
        }
        n265 = shared-variable ".\\local SCA shared var lib.lvlib\\Sample Rod Bypass"() -> (w560:bool)  [unwired: 1 in, 1 out]
        n266 = shared-variable "SCA-cRIO\\global SCA shared var lib.lvlib\\Sample Rod status"(error in=w563) -> (w561:T5)  [unwired: 1 out]
        n267 = Select(t=Vertical_Rod_states."rod up" ("y"), s=w560, f=w561) -> (s? t:f=w559:T5)
        n268 = case shown="\"rod up\"" w559 {
          tunnel: w558 -> [w575 w581]
          tunnel: w557 -> [w574 w580]
          tunnel: w556 -> [w573 _]
          tunnel: [w569 "sample rod up" ("Status Message")] -> w554
          tunnel: [w570 w578] -> w553
          tunnel: [w571 w577] -> w552
          tunnel: [w572 w576] -> w551
          frame "status unclear", "rod down", Default {
            n269 = shared-variable ".\\global SCA shared var lib.lvlib\\Sample Rod Timeout"() -> (w568:u32)  [unwired: 1 in, 1 out]
            n270 = call "SCA state Transition Timeout Check.vi"("Start Time"=w573, "Timeout limit"=w568, "Current State In"=w574, "Modified Array of states in"=w575) -> ("Status Message"=w569:string, "millisecond timer value out"=w570:u32, "Next State"=w571:T7, "Modified Array of states out"=w572:T7[])  [unwired: 4 in]
          }
          frame "rod up" {
            n271 = call "Modify array of SCA states.vi"("Current State"=w580, "Array of states to process"=w581) -> ("Next State"=w577:T7, "Modified Array of states"=w576:T7[])  [unwired: 7 in]
            n272 = Tick Count (ms)() -> (millisecond timer value=w578:u32)
          }
        }
      }
      frame "sample rod down" {
        n273 = shared-variable "SCA-cRIO\\global SCA shared var lib.lvlib\\Retract Rod Status"() -> (w600:T4)  [unwired: 1 in, 1 out]
        n274 = shared-variable "SCA-cRIO\\global SCA shared var lib.lvlib\\Insert Rod Status"() -> (w598:T4)  [unwired: 1 in, 1 out]
        n275 = shared-variable ".\\local SCA shared var lib.lvlib\\Retract Rod Bypass"() -> (w594:bool)  [unwired: 1 in, 1 out]
        n276 = shared-variable ".\\local SCA shared var lib.lvlib\\Insert Rod Bypass"() -> (w596:bool)  [unwired: 1 in, 1 out]
        n277 = Equal?(x=w598, y=Horizontal_Rod_states."rod out" ("Enum")) -> (x = y?=w597:bool)
        n278 = Equal?(x=w600, y=Horizontal_Rod_states."rod out" ("Enum")) -> (x = y?=w595:bool)
        n279 = Or(x=w596, y=w597) -> (x .or. y?=w593:bool)
        n280 = Or(x=w594, y=w595) -> (x .or. y?=w592:bool)
        n281 = Build Array(w593, w592) -> (w590:bool[])
        n282 = And Array Elements(Boolean array=w590) -> (logical AND=w591:bool)
        n283 = case shown="True" w591 {
          tunnel: w590 -> [w609 _]
          tunnel: w589 -> [w605 w625]
          tunnel: w588 -> [_ w624]
          tunnel: w587 -> [_ w623]
          tunnel: ["sample rod down interlocks not satisfied" ("Status Message") w622] -> w586
          tunnel: [w602 w621] -> w584
          tunnel: [w603 w620] -> w583
          tunnel: [w604 w619] -> w582
          frame False {
            n284 = Search 1D Array(1D array=w609, element=FALSE) -> (index of element=w607:i32)  [unwired: 1 in]
            n285 = case shown="0, Default" w607 {
              tunnel: w605 -> [w610 w617]
              tunnel: [w612 w615] -> w604
              tunnel: [w611 w614] -> w603
              frame 0, Default {
                w611 = SCA_states."insert rod out" ("SC2 state")
                n286 = Insert Into Array(array=w610, index=0, new element=w611) -> (w612:T7[])
              }
              frame 1 {
                w614 = SCA_states."retract rod out" ("SC2 state")
                n287 = Insert Into Array(array=w617, index=0, new element=w614) -> (w615:T7[])
              }
            }
            n288 = Tick Count (ms)() -> (millisecond timer value=w602:u32)
          }
          frame True {
            n289 = shared-variable "SCA-cRIO\\Mod8\\Sample Rod Actuator"(TRUE ("sc gate valve")) -> (error out=w628:errorcluster)  [unwired: 1 in]
            n290 = shared-variable ".\\local SCA shared var lib.lvlib\\Sample Rod Bypass"() -> (w630:bool)  [unwired: 1 in, 1 out]
            n291 = shared-variable "SCA-cRIO\\global SCA shared var lib.lvlib\\Sample Rod status"(error in=w628) -> (w627:T5)  [unwired: 1 out]
            n292 = Select(t=Vertical_Rod_states."rod up" ("y"), s=w630, f=w627) -> (s? t:f=w626:T5)
            n293 = case shown="\"status unclear\", \"rod up\", Default" w626 {
              tunnel: w623 -> [w637 _]
              tunnel: w625 -> [w636 w644]
              tunnel: w624 -> [w635 w643]
              tunnel: [w634 w642] -> w619
              tunnel: [w633 w641] -> w620
              tunnel: [w632 w640] -> w621
              tunnel: [w631 "sample rod down" ("Status Message")] -> w622
              frame "status unclear", "rod up", Default {
                n294 = shared-variable ".\\global SCA shared var lib.lvlib\\Sample Rod Timeout"() -> (w638:u32)  [unwired: 1 in, 1 out]
                n295 = call "SCA state Transition Timeout Check.vi"("Start Time"=w637, "Timeout limit"=w638, "Current State In"=w635, "Modified Array of states in"=w636) -> ("Status Message"=w631:string, "millisecond timer value out"=w632:u32, "Next State"=w633:T7, "Modified Array of states out"=w634:T7[])  [unwired: 4 in]
              }
              frame "rod down" {
                n296 = call "Modify array of SCA states.vi"("Current State"=w643, "Array of states to process"=w644) -> ("Next State"=w641:T7, "Modified Array of states"=w642:T7[])  [unwired: 7 in]
                n297 = Tick Count (ms)() -> (millisecond timer value=w640:u32)
              }
            }
          }
        }
      }
      frame "retract rod in" {
        n298 = shared-variable "SCA-cRIO\\global SCA shared var lib.lvlib\\Sample Rod status"() -> (w649:T5)  [unwired: 1 in, 1 out]
        n299 = shared-variable "SCA-cRIO\\global SCA shared var lib.lvlib\\Insert Rod Status"() -> (w667:T4)  [unwired: 1 in, 1 out]
        n300 = shared-variable "SCA-cRIO\\global SCA shared var lib.lvlib\\Wheel GV Status"() -> (w669:enum16{"status unclear", "closed", "open"})  [unwired: 1 in, 1 out]
        n301 = shared-variable ".\\local SCA shared var lib.lvlib\\Wheel GV Bypass"() -> (w663:bool)  [unwired: 1 in, 1 out]
        n302 = shared-variable ".\\local SCA shared var lib.lvlib\\Sample Rod Bypass"() -> (w647:bool)  [unwired: 1 in, 1 out]
        n303 = shared-variable ".\\local SCA shared var lib.lvlib\\Insert Rod Bypass"() -> (w665:bool)  [unwired: 1 in, 1 out]
        n304 = Equal?(x=w667, y=Horizontal_Rod_states."rod out" ("Enum")) -> (x = y?=w666:bool)
        n305 = Equal?(x=w669, y=enum16{"status unclear", "closed", "open"}."open") -> (x = y?=w664:bool)
        n306 = Equal?(x=w649, y=Vertical_Rod_states."rod up") -> (x = y?=w648:bool)
        n307 = Or(x=w665, y=w666) -> (x .or. y?=w662:bool)
        n308 = Or(x=w663, y=w664) -> (x .or. y?=w661:bool)
        n309 = Or(x=w647, y=w648) -> (x .or. y?=w646:bool)
        n310 = Build Array(w662, w661, w646) -> (w659:bool[])
        n311 = And Array Elements(Boolean array=w659) -> (logical AND=w660:bool)
        n312 = case shown="True" w660 {
          tunnel: w659 -> [w677 _]
          tunnel: w658 -> [w673 w697]
          tunnel: w657 -> [_ w696]
          tunnel: w656 -> [_ w695]
          tunnel: ["retract rod in interlocks not satisfied" ("Status Message") w694] -> w654
          tunnel: [w670 w693] -> w653
          tunnel: [w671 w692] -> w652
          tunnel: [w672 w691] -> w651
          frame False {
            n313 = Search 1D Array(1D array=w677, element=FALSE) -> (index of element=w675:i32)  [unwired: 1 in]
            n314 = case shown="1" w675 {
              tunnel: w673 -> [w678 w685 w689]
              tunnel: [w680 w683 w687] -> w672
              tunnel: [w679 w682 w686] -> w671
              frame 0, Default {
                w679 = SCA_states."insert rod out" ("SC2 state")
                n315 = Insert Into Array(array=w678, index=0, new element=w679) -> (w680:T7[])
              }
              frame 1 {
                w682 = SCA_states."wheel GV open" ("SC2 state")
                n316 = Insert Into Array(array=w685, index=0, new element=w682) -> (w683:T7[])
              }
              frame 2 {
                w686 = SCA_states."sample rod up" ("SC2 state")
                n317 = Insert Into Array(array=w689, index=0, new element=w686) -> (w687:T7[])
              }
            }
            n318 = Tick Count (ms)() -> (millisecond timer value=w670:u32)
          }
          frame True {
            n319 = shared-variable "SCA-cRIO\\Mod8\\Retract Rod Actuator"(TRUE ("sc gate valve")) -> (error out=w700:errorcluster)  [unwired: 1 in]
            n320 = shared-variable ".\\local SCA shared var lib.lvlib\\Retract Rod Bypass"() -> (w702:bool)  [unwired: 1 in, 1 out]
            n321 = shared-variable "SCA-cRIO\\global SCA shared var lib.lvlib\\Retract Rod Status"(error in=w700) -> (w699:T4)  [unwired: 1 out]
            n322 = Select(t=Horizontal_Rod_states."rod in", s=w702, f=w699) -> (s? t:f=w698:T4)
            n323 = case shown="\"rod in\"" w698 {
              tunnel: w695 -> [w709 _]
              tunnel: w697 -> [w708 w716]
              tunnel: w696 -> [w707 w715]
              tunnel: [w706 w714] -> w691
              tunnel: [w705 w713] -> w692
              tunnel: [w704 w712] -> w693
              tunnel: [w703 "retract rod in" ("Status Message")] -> w694
              frame "status unclear", "rod out", Default {
                n324 = shared-variable ".\\global SCA shared var lib.lvlib\\Retract Rod Timeout"() -> (w710:u32)  [unwired: 1 in, 1 out]
                n325 = call "SCA state Transition Timeout Check.vi"("Start Time"=w709, "Timeout limit"=w710, "Current State In"=w707, "Modified Array of states in"=w708) -> ("Status Message"=w703:string, "millisecond timer value out"=w704:u32, "Next State"=w705:T7, "Modified Array of states out"=w706:T7[])  [unwired: 4 in]
              }
              frame "rod in" {
                n326 = call "Modify array of SCA states.vi"("Current State"=w715, "Array of states to process"=w716) -> ("Next State"=w713:T7, "Modified Array of states"=w714:T7[])  [unwired: 7 in]
                n327 = Tick Count (ms)() -> (millisecond timer value=w712:u32)
              }
            }
          }
        }
      }
      frame "retract rod out" {
        n328 = flat-sequence {
          tunnel: [w731] -> w717
          tunnel: [w734] -> w730
          tunnel: w717 -> [w734]
          frame #0 {
            n329 = shared-variable "SCA-cRIO\\Mod8\\Retract Rod Actuator"(FALSE ("Sample Rod Actuator")) -> (error out=w731:errorcluster)  [unwired: 1 in]
          }
          frame #1 {
            n330 = Wait (ms)(milliseconds to wait=u32 500) -> ()  [unwired: 1 out]
          }
        }
        n331 = shared-variable ".\\local SCA shared var lib.lvlib\\Retract Rod Bypass"() -> (w729:bool)  [unwired: 1 in, 1 out]
        n332 = shared-variable "SCA-cRIO\\global SCA shared var lib.lvlib\\Retract Rod Status"(error in=w730) -> (w727:T4)  [unwired: 1 out]
        n333 = Select(t=Horizontal_Rod_states."rod out" ("Enum"), s=w729, f=w727) -> (s? t:f=w726:T4)
        n334 = case shown="\"rod out\"" w726 {
          tunnel: w725 -> [w741 w748]
          tunnel: w724 -> [w740 w747]
          tunnel: w723 -> [w739 _]
          tunnel: [w735 "retract rod out" ("Status Message")] -> w721
          tunnel: [w738 w745] -> w720
          tunnel: [w737 w744] -> w719
          tunnel: [w736 w743] -> w718
          frame "status unclear", "rod in", Default {
            n335 = shared-variable ".\\global SCA shared var lib.lvlib\\Retract Rod Timeout"() -> (w742:u32)  [unwired: 1 in, 1 out]
            n336 = call "SCA state Transition Timeout Check.vi"("Start Time"=w739, "Timeout limit"=w742, "Current State In"=w740, "Modified Array of states in"=w741) -> ("Status Message"=w735:string, "millisecond timer value out"=w738:u32, "Next State"=w737:T7, "Modified Array of states out"=w736:T7[])  [unwired: 4 in]
          }
          frame "rod out" {
            n337 = call "Modify array of SCA states.vi"("Current State"=w747, "Array of states to process"=w748) -> ("Next State"=w744:T7, "Modified Array of states"=w743:T7[])  [unwired: 7 in]
            n338 = Tick Count (ms)() -> (millisecond timer value=w745:u32)
          }
        }
      }
      frame "insert rod in" {
        n339 = shared-variable "SCA-cRIO\\global SCA shared var lib.lvlib\\Retract Rod Status"() -> (w771:T4)  [unwired: 1 in, 1 out]
        n340 = shared-variable "SCA-cRIO\\global SCA shared var lib.lvlib\\Sample Rod status"() -> (w761:T5)  [unwired: 1 in, 1 out]
        n341 = shared-variable "SCA-cRIO\\global SCA shared var lib.lvlib\\Wheel GV Status"() -> (w773:enum16{"status unclear", "closed", "open"})  [unwired: 1 in, 1 out]
        n342 = shared-variable ".\\local SCA shared var lib.lvlib\\Wheel GV Bypass"() -> (w767:bool)  [unwired: 1 in, 1 out]
        n343 = shared-variable ".\\local SCA shared var lib.lvlib\\Sample Rod Bypass"() -> (w759:bool)  [unwired: 1 in, 1 out]
        n344 = shared-variable ".\\local SCA shared var lib.lvlib\\Retract Rod Bypass"() -> (w769:bool)  [unwired: 1 in, 1 out]
        n345 = Equal?(x=w771, y=Horizontal_Rod_states."rod out" ("Enum")) -> (x = y?=w770:bool)
        n346 = Equal?(x=w773, y=enum16{"status unclear", "closed", "open"}."open") -> (x = y?=w768:bool)
        n347 = Equal?(x=w761, y=Vertical_Rod_states."rod up") -> (x = y?=w760:bool)
        n348 = Or(x=w769, y=w770) -> (x .or. y?=w766:bool)
        n349 = Or(x=w767, y=w768) -> (x .or. y?=w765:bool)
        n350 = Or(x=w759, y=w760) -> (x .or. y?=w758:bool)
        n351 = Build Array(w766, w765, w758) -> (w763:bool[])
        n352 = And Array Elements(Boolean array=w763) -> (logical AND=w764:bool)
        n353 = case shown="True" w764 {
          tunnel: w763 -> [w781 _]
          tunnel: w756 -> [w777 w801]
          tunnel: w755 -> [_ w800]
          tunnel: w754 -> [_ w799]
          tunnel: ["retract rod in interlocks not satisfied" ("Status Message") w798] -> w753
          tunnel: [w774 w797] -> w749
          tunnel: [w775 w796] -> w750
          tunnel: [w776 w795] -> w751
          frame False {
            n354 = Search 1D Array(1D array=w781, element=FALSE) -> (index of element=w779:i32)  [unwired: 1 in]
            n355 = case shown="2" w779 {
              tunnel: w777 -> [w782 w789 w793]
              tunnel: [w784 w787 w791] -> w776
              tunnel: [w783 w786 w790] -> w775
              frame 0, Default {
                w783 = SCA_states."retract rod out" ("SC2 state")
                n356 = Insert Into Array(array=w782, index=0, new element=w783) -> (w784:T7[])
              }
              frame 1 {
                w786 = SCA_states."wheel GV open" ("SC2 state")
                n357 = Insert Into Array(array=w789, index=0, new element=w786) -> (w787:T7[])
              }
              frame 2 {
                w790 = SCA_states."sample rod up" ("SC2 state")
                n358 = Insert Into Array(array=w793, index=0, new element=w790) -> (w791:T7[])
              }
            }
            n359 = Tick Count (ms)() -> (millisecond timer value=w774:u32)
          }
          frame True {
            n360 = shared-variable "SCA-cRIO\\Mod8\\Insert Rod Actuator"(TRUE ("sc gate valve")) -> (error out=w804:errorcluster)  [unwired: 1 in]
            n361 = shared-variable ".\\local SCA shared var lib.lvlib\\Insert Rod Bypass"() -> (w806:bool)  [unwired: 1 in, 1 out]
            n362 = shared-variable "SCA-cRIO\\global SCA shared var lib.lvlib\\Insert Rod Status"(error in=w804) -> (w803:T4)  [unwired: 1 out]
            n363 = Select(t=Horizontal_Rod_states."rod in", s=w806, f=w803) -> (s? t:f=w802:T4)
            n364 = case shown="\"status unclear\", \"rod out\", Default" w802 {
              tunnel: w799 -> [w813 _]
              tunnel: w801 -> [w812 w820]
              tunnel: w800 -> [w811 w819]
              tunnel: [w810 w818] -> w795
              tunnel: [w809 w817] -> w796
              tunnel: [w808 w816] -> w797
              tunnel: [w807 "insert rod in" ("Status Message")] -> w798
              frame "status unclear", "rod out", Default {
                n365 = shared-variable ".\\global SCA shared var lib.lvlib\\Insert Rod Timeout"() -> (w814:u32)  [unwired: 1 in, 1 out]
                n366 = call "SCA state Transition Timeout Check.vi"("Start Time"=w813, "Timeout limit"=w814, "Current State In"=w811, "Modified Array of states in"=w812) -> ("Status Message"=w807:string, "millisecond timer value out"=w808:u32, "Next State"=w809:T7, "Modified Array of states out"=w810:T7[])  [unwired: 4 in]
              }
              frame "rod in" {
                n367 = call "Modify array of SCA states.vi"("Current State"=w819, "Array of states to process"=w820) -> ("Next State"=w817:T7, "Modified Array of states"=w818:T7[])  [unwired: 7 in]
                n368 = Tick Count (ms)() -> (millisecond timer value=w816:u32)
              }
            }
          }
        }
      }
      frame "insert rod out" {
        n369 = flat-sequence {
          tunnel: [w835] -> w821
          tunnel: [w838] -> w834
          tunnel: w821 -> [w838]
          frame #0 {
            n370 = shared-variable "SCA-cRIO\\Mod8\\Insert Rod Actuator"(FALSE ("Sample Rod Actuator")) -> (error out=w835:errorcluster)  [unwired: 1 in]
          }
          frame #1 {
            n371 = Wait (ms)(milliseconds to wait=u32 500) -> ()  [unwired: 1 out]
          }
        }
        n372 = shared-variable ".\\local SCA shared var lib.lvlib\\Insert Rod Bypass"() -> (w833:bool)  [unwired: 1 in, 1 out]
        n373 = shared-variable "SCA-cRIO\\global SCA shared var lib.lvlib\\Insert Rod Status"(error in=w834) -> (w822:T4)  [unwired: 1 out]
        n374 = Select(t=Horizontal_Rod_states."rod out" ("Enum"), s=w833, f=w822) -> (s? t:f=w831:T4)
        n375 = case shown="\"status unclear\", \"rod in\", Default" w831 {
          tunnel: w830 -> [w845 w852]
          tunnel: w829 -> [w844 w851]
          tunnel: w828 -> [w843 _]
          tunnel: [w839 "insert rod out" ("Status Message")] -> w823
          tunnel: [w842 w849] -> w826
          tunnel: [w841 w848] -> w825
          tunnel: [w840 w847] -> w824
          frame "status unclear", "rod in", Default {
            n376 = shared-variable ".\\global SCA shared var lib.lvlib\\Insert Rod Timeout"() -> (w846:u32)  [unwired: 1 in, 1 out]
            n377 = call "SCA state Transition Timeout Check.vi"("Start Time"=w843, "Timeout limit"=w846, "Current State In"=w844, "Modified Array of states in"=w845) -> ("Status Message"=w839:string, "millisecond timer value out"=w842:u32, "Next State"=w841:T7, "Modified Array of states out"=w840:T7[])  [unwired: 4 in]
          }
          frame "rod out" {
            n378 = call "Modify array of SCA states.vi"("Current State"=w851, "Array of states to process"=w852) -> ("Next State"=w848:T7, "Modified Array of states"=w847:T7[])  [unwired: 7 in]
            n379 = Tick Count (ms)() -> (millisecond timer value=w849:u32)
          }
        }
      }
      frame "change sample start" {
        n380 = call "Modify array of SCA states.vi"("Current State"=w856, "Array of states to process"=w858) -> ("Next State"=w855:T7, "Modified Array of states"=w857:T7[])  [unwired: 7 in]
        n381 = shared-variable ".\\global SCA shared var lib.lvlib\\SCA status"(SCA_broadcast_status."Changing samples" ("SCA status")) -> ()  [unwired: 1 in, 1 out]
        n382 = Tick Count (ms)() -> (millisecond timer value=w859:u32)
      }
      frame "rotate wheel" {
        # "Slow down for short moves"
        # "in motor steps"
        # "The counter logic here (along with \"wait position\") doesn't appear to have a clear purpose.  Doesn't appear that the failure state could ever be acheived as the max timer"
        n383 = local read "New Move"() -> (w860:dbl)
        n384 = shared-variable ".\\local SCA shared var lib.lvlib\\Motor Status"(FALSE ("Motor Status")) -> (error out=w869:errorcluster)  [unwired: 1 in]
        n385 = Absolute Value(x=w860) -> (abs(x)=w867:dbl)
        n386 = shared-variable ".\\local SCA shared var lib.lvlib\\Execute Move"(error in=w869) -> (w873:bool)  [unwired: 1 out]
        n387 = Less?(x=w867, y=100.0) -> (x < y?=w865:bool)
        n388 = case shown="True" w865 {
          tunnel: [w880 10.0] -> w864
          tunnel: [w880 100.0] -> w863
          frame False {
            w880 = 10000.0
          }
          frame True {
          }
        }
        n389 = xnode "Straight-Line Move"("resource"=w879, "execute"=w873, "position"=w860, "velocity"=w864, "acceleration"=w864, "deceleration"=w864, "accel. jerk"=w863, "decel. jerk"=w863) -> ("error out"=→"Rotate Wheel error":errorcluster, "done"=w861:bool)  [unwired: 1 in, 1 out]
        "Rotation done" <- w861
        n390 = Not(x=w861) -> (.not. x?=w870:bool)
        n391 = shared-variable ".\\local SCA shared var lib.lvlib\\Execute Move"(w870) -> ()  [unwired: 1 in, 1 out]
        n392 = Select(t=SCA_states."check position" ("SC2 state"), s=w861, f=SCA_states."rotate wheel" ("SC2 state")) -> (s? t:f=w871:T7)
      }
      frame "check position" {
        n393 = Tick Count (ms)() -> (millisecond timer value=w903:u32)
        n394 = shared-variable ".\\global SCA shared var lib.lvlib\\Rotate Wheel timeout"() -> (w908:u32)  [unwired: 1 in, 1 out]
        n395 = shared-variable ".\\global SCA shared var lib.lvlib\\Rotate Wheel Minimum Time"() -> (w905:u32)  [unwired: 1 in, 1 out]
        n396 = Subtract(x=w903, y=w906) -> (x-y=w907:u32)
        n397 = Greater?(x=w908, y=w907) -> (0:w900:bool)
        n398 = Subtract(x=w903, y=w909) -> (x-y=w904:u32)
        n399 = Less?(x=w905, y=w904) -> (x < y?=w902:bool)
        n400 = And(x=w900, y=w902) -> (x .and. y?=w901:bool)
        n401 = case shown="True" w901 {
          tunnel: w917 -> [w924 w978]
          tunnel: [w920 w977] -> w916
          tunnel: [w918 w976] -> w915
          tunnel: [w923 w975] -> w914
          tunnel: w913 -> [_ w974]
          tunnel: w912 -> [w925 w973]
          tunnel: [w922 w972] -> w911
          tunnel: [w926 w971] -> w910
          tunnel: w909 -> [w919 w970]
          tunnel: w906 -> [w921 w969]
          tunnel: w900 -> [w927 _]
          frame False {
            n402 = case shown="True" w927 {
              tunnel: [w939 "waiting to check position"] -> w926
              tunnel: w925 -> [w933 w955]
              tunnel: w924 -> [w934 w956]
              tunnel: [w938 w956] -> w923
              tunnel: [w937 w955] -> w922
              tunnel: w921 -> [w931 w954]
              tunnel: [w932 w954] -> w920
              tunnel: w919 -> [w930 w953]
              tunnel: [w929 w953] -> w918
              frame False {
                # "Timeout reached"
                n403 = local read "Step Window Radius"() -> (w928:u8)
                n404 = Less?(x=w928, y=u8 2) -> (x < y?=w935:bool)
                n405 = case shown="False" w935 {
                  tunnel: ["Wheel rotation timed out" "relaxing precision of wheel rotation"] -> w939
                  tunnel: [SCA_states."wait" ("SC2 state") w951] -> w938
                  tunnel: [w943 w950] -> w937
                  tunnel: w934 -> [_ w951]
                  tunnel: w933 -> [_ w950]
                  tunnel: w928 -> [_ w949]
                  tunnel: [w942 w948] -> w932
                  tunnel: w931 -> [w942 _]
                  tunnel: w930 -> [w941 w947]
                  tunnel: [w941 w947] -> w929
                  frame False {
                    w943 = T7[] [enum."wait"] items=["initialize", "wait", "change sample start", "change sample", "check position", "rotate wheel", "sample change complete", "sample rod up", "sample rod down", "retract rod in", "retract rod out", "insert rod in", "insert rod out", "wheel GV open", "wheel GV close", "vent source", "pump source", "shutdown"]
                    n406 = shared-variable ".\\local SCA shared var lib.lvlib\\Motor Status"(TRUE ("Motor Status")) -> ()  [unwired: 1 in, 1 out]
                  }
                  frame True {
                    # "Add extra step to window radius"
                    n407 = Tick Count (ms)() -> (millisecond timer value=w948:u32)
                    n408 = Increment(x=w949) -> (x+1=w946:u8)
                    n409 = local write "Step Window Radius"(w946) -> ()
                  }
                }
              }
              frame True {
                # "Haven't met minimum wait time yet"
              }
            }
          }
          frame True {
            # "For long moves, shift \ntarget position"
            # "14-bit encoder # steps"
            # "Motor steps per revolution"
            # "Move in motor steps"
            n410 = local read "Encoder position"() -> (w958:u16)
            n411 = call "SCA Sample-Encoder conversion.vi"("Step Window Radius"="Step Window Radius", "Rollover Sample"="Rollover Sample", "Encoder Offset"="Encoder Offset", "Encoder Position"=w958, "Desired Sample"="New sample") -> ("Window limit 1"=→"Window Limit 1":i16, "Within Range?"=w979:bool, "Encoder destination"=w988:i16, "Window limit 2"=→"Window Limit 2":i16, "New move (encoder steps)"=w984:i16)  [unwired: 2 in]
            "Encoder Destination" <- w988
            "In Range?" <- w979
            n412 = To Double Precision Float(number=w984) -> (double precision float=w980:dbl)
            n413 = Divide(x=50000.0, y=16384.0) -> (x/y=w983:dbl)
            n414 = shared-variable "SCA-cRIO\\global SCA shared var lib.lvlib\\Encoder Destination"(w988) -> ()  [unwired: 1 in, 1 out]
            n415 = shared-variable ".\\local SCA shared var lib.lvlib\\Motor Status"(w979) -> ()  [unwired: 1 in, 1 out]
            n416 = Multiply(x=w983, y=w980) -> (x*y=w989:dbl)
            n417 = Round To Nearest(number=w989) -> (nearest integer value=w963:dbl)
            n418 = Absolute Value(x=w963) -> (abs(x)=w962:dbl)
            n419 = Less?(x=w962, y=100.0) -> (x < y?=w965:bool)
            n420 = case shown="True" w979 {
              tunnel: [SCA_states."rotate wheel" ("SC2 state") w1002] -> w975
              tunnel: ["rotating sample wheel" "rotation complete"] -> w971
              tunnel: [w990 w1001] -> w972
              tunnel: [w991 w995] -> w976
              tunnel: [w992 w995] -> w977
              tunnel: w970 -> [_ _]
              tunnel: w969 -> [w992 _]
              tunnel: w978 -> [_ w1000]
              tunnel: w973 -> [w990 w999]
              tunnel: w974 -> [_ w997]
              frame False {
                # "wheel not in correct position, rotate again"
                n421 = Tick Count (ms)() -> (millisecond timer value=w991:u32)
              }
              frame True {
                n422 = call "Modify array of SCA states.vi"("Current State"=w1000, "Array of states to process"=w999) -> ("Next State"=w1002:T7, "Modified Array of states"=w1001:T7[])  [unwired: 7 in]
                n423 = xnode "Straight-Line Move"("resource"=w997, "execute"=FALSE) -> ()  [unwired: 8 in, 6 out]
                n424 = Tick Count (ms)() -> (millisecond timer value=w995:u32)
              }
            }
            n425 = Subtract(x=w963, y=10.0) -> (x-y=w967:dbl)
            n426 = Select(t=w963, s=w965, f=w967) -> (s? t:f=w968:dbl)
            "New Move" <- w968
            n427 = shared-variable "SCA-cRIO\\global SCA shared var lib.lvlib\\New Move"(w968) -> ()  [unwired: 1 in, 1 out]
          }
        }
      }
      frame "sample change complete" {
        n428 = shared-variable "SCA-cRIO\\global SCA shared var lib.lvlib\\Step Window Radius"() -> (w1029:u8)  [unwired: 1 in, 1 out]
        n429 = call "Modify array of SCA states.vi"("Current State"=w1034, "Array of states to process"=w1035) -> ("Next State"=w1032:T7, "Modified Array of states"=w1033:T7[])  [unwired: 7 in]
        n430 = shared-variable ".\\global SCA shared var lib.lvlib\\SCA status"(SCA_broadcast_status."Sample change complete" ("Changing Sample")) -> (error out=w1036:errorcluster)  [unwired: 1 in]
        n431 = Tick Count (ms)() -> (millisecond timer value=w1038:u32)
        n432 = local write "Step Window Radius"(w1029) -> ()
        n433 = shared-variable ".\\local SCA shared var lib.lvlib\\Motor Status"(TRUE ("Motor Status"), error in=w1036) -> ()  [unwired: 1 out]
      }
    }
    "action" <- w403
    "SCA next state" <- w401
    n434 = shared-variable "SCA-cRIO\\global SCA shared var lib.lvlib\\Status Message"(w406) -> ()  [unwired: 1 in, 1 out]
    n435 = call "Wait Until Next Multiple"("Count(mSec)"=u32 5) -> ()  [unwired: 1 out]
  }
  n436 = node-c288(w7) -> ()  [unwired: 1 out]
